vi "main OP300.vi"() -> ()   [LabVIEW 2020]
uses:
  SubVI/OP300ZP_state.ctl
  <userlib>/Alex.vi/FGV.ctl
  <vilib>/QMT/GDataBase for MySQL(tm)/MySQL/public/controls/DateType.ctl
  Documents/GitHub/ZEN-PLUS/OP500/VG/VG_progressBar.vi
  SubVI/CheminDeBase.vi
  <vilib>/Utility/error.llb/Error Cluster From Error Code.vi
  VG/PN.vi
  VG/IS30%.vi
  VG/R.vi
  VG/VG_BT3562.vi
  OP500/VG/VG_ST5520.vi
  Documents/GitHub/ZEN-PLUS/OP300/EN PRODUCTION/OP300-CONTI-AUTO/VG/VG_ARDUINO.vi
  SubVI/VG_HYDRAU.vi
  VG/VG_MX5060.vi
  <vilib>/QMT/GDataBase for MySQL(tm)/MySQL/MySQLConnector.lvclass
panel:
  out "chaîne concaténée":string
  out "MX5060":refnum<visa-resource-name>
  out "ST5520":refnum<visa-resource-name>
  out "Revision":i32=334
  in  "arrêt":bool
  out "BT3562":refnum<visa-resource-name>
  out "Application Directory":path caption="Chemin programme"
  out "Compt":i32
  in  "DERNIER2":bool
  in  "last?":bool
  out "Cluster 2":T1
  out "IS30% ?":bool
  out "BDD":T2
  out "VISA OUT":T3
  out "progression":dbl(slide) scale=0.0..60.0
  out "PN":string
  out "errout":errorcluster={"status"=TRUE, "code"=0, "source"="PCAN_CHANNEL ILLEGAL"}
  out "errout":errorcluster caption="sortie d'erreur"
  out "STOP":bool
  out "TOP":string
  out "DRAW":picture
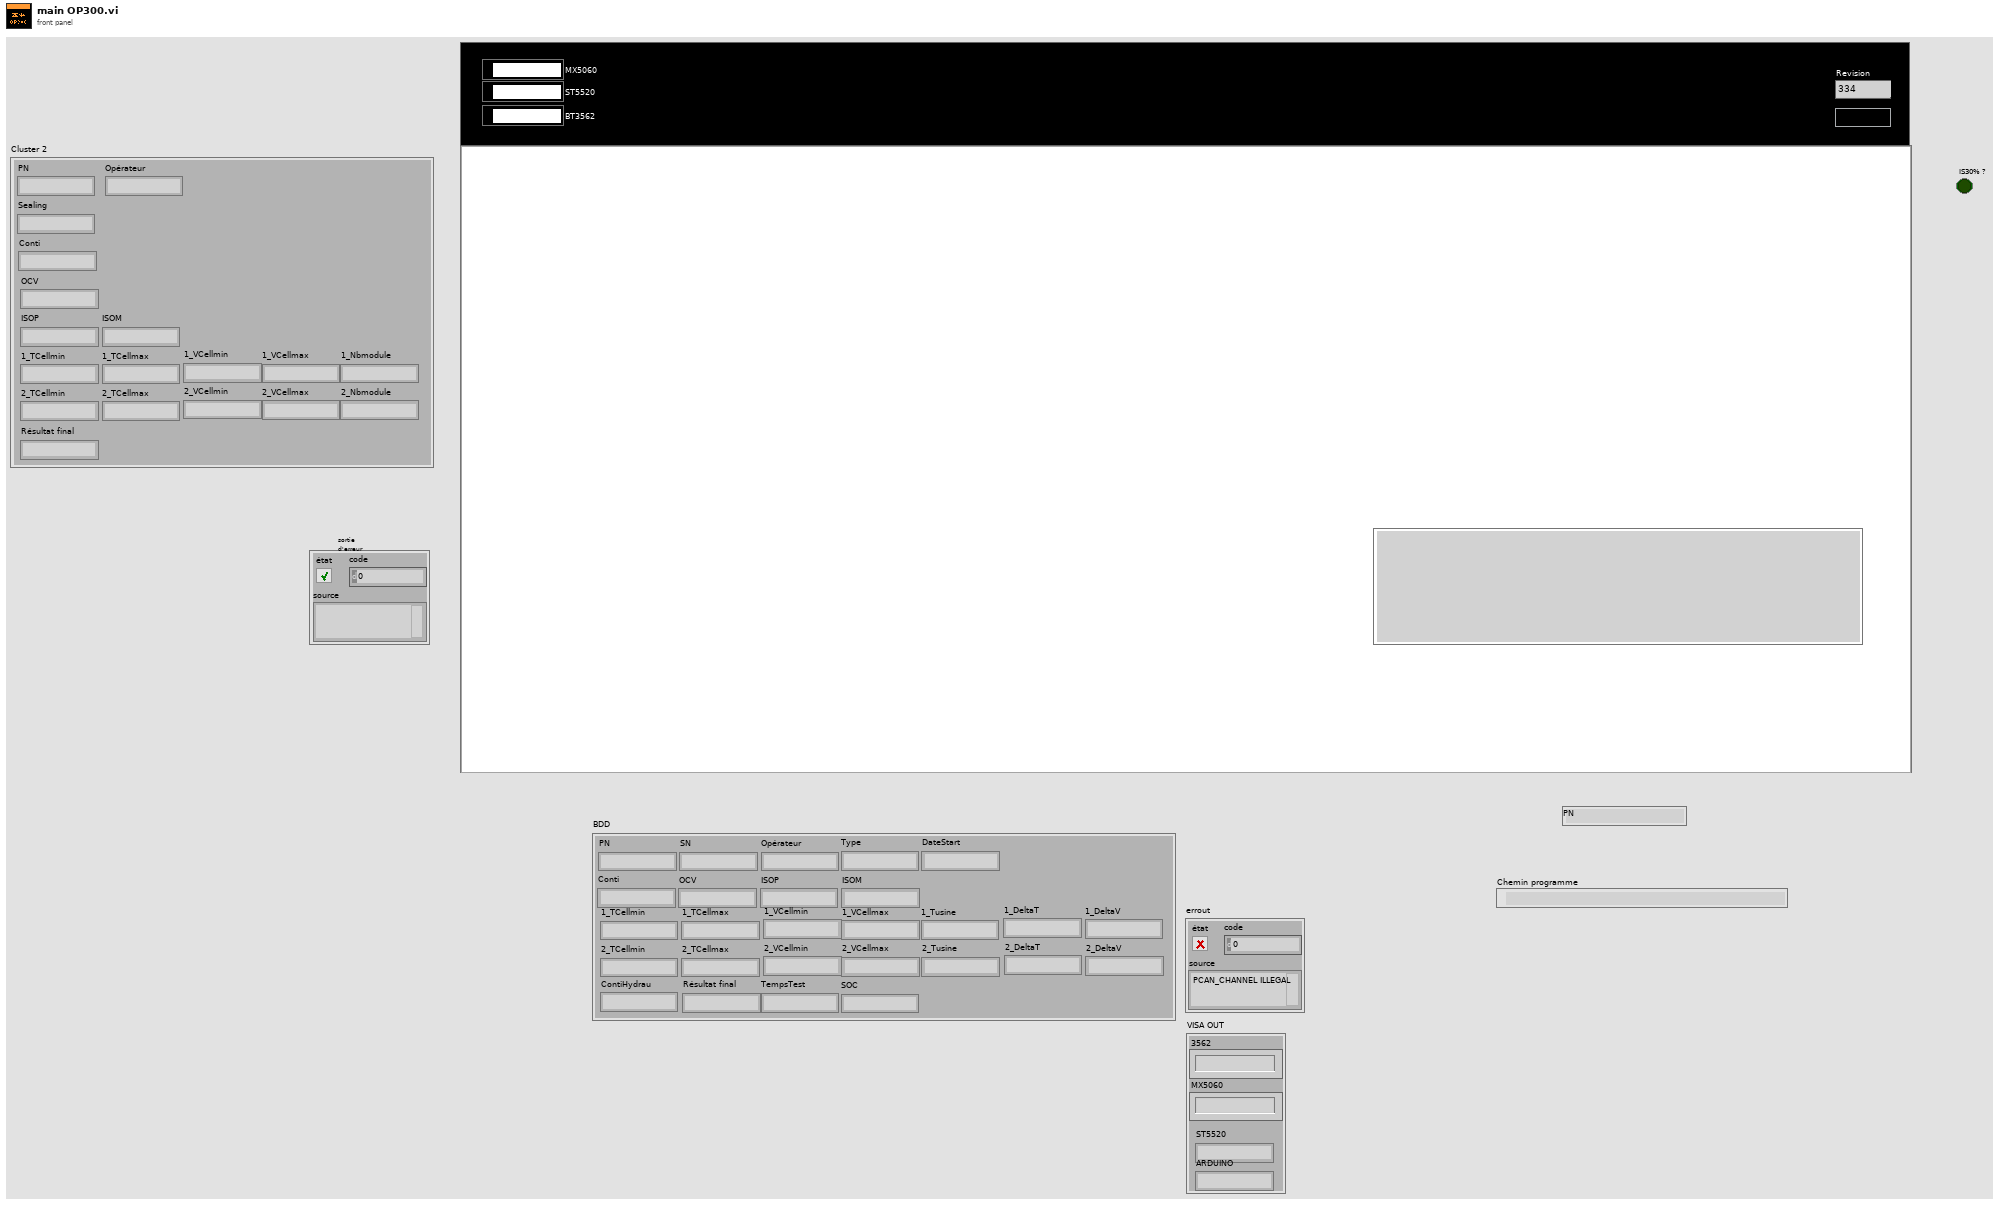
[diagram p1: front panel]
types:
  T1 = cluster{"PN":string, "Opérateur":string, "Sealing":string, "Conti":string, "OCV":string, "ISOP":string, "ISOM":string, "1_TCellmin":string, "1_TCellmax":string, "1_VCellmin":string, "1_VCellmax":string, "1_Nbmodule":string, "2_TCellmin":string, "2_TCellmax":string, "2_VCellmin":string, "2_VCellmax":string, "2_Nbmodule":string, "Résultat final":string}
  T2 = cluster{"PN":string, "SN":string, "Opérateur":string, "Type":string, "DateStart":string, "Conti":string, "OCV":string, "ISOP":string, "ISOM":string, "1_TCellmin":string, "1_TCellmax":string, "1_VCellmin":string, "1_VCellmax":string, "1_Tusine":string, "1_DeltaT":string, "1_DeltaV":string, "2_TCellmin":string, "2_TCellmax":string, "2_VCellmin":string, "2_VCellmax":string, "2_Tusine":string, "2_DeltaT":string, "2_DeltaV":string, "ContiHydrau":string, "Résultat final":string, "TempsTest":string, "SOC":string}
  T3 = cluster{"3562":string, "MX5060":string, "ST5520":string, "ARDUINO":string}
  T4 = cluster{"PN":string, "Sealing":string, "Opérateur":string, "Conti":string, "OCV":string, "ISOP":string, "ISOM":string, "1_TCellmin":string, "1_TCellmax":string, "1_VCellmin":string, "1_VCellmax":string, "1_Nbmodule":string, "2_TCellmin":string, "2_TCellmax":string, "2_VCellmin":string, "2_VCellmax":string, "2_Nbmodule":string, "Résultat final":string, "2_Nbmodule 2":string, "2_VCellmax 2":string, "2_VCellmin 2":string, "2_TCellmax 2":string, "2_TCellmin 2":string, "1_Nbmodule 2":string, "1_VCellmax 2":string, "1_VCellmin 2":string, "1_TCellmax 2":string}
  T5 = cluster{"3562":string, "MX5060":string, "ST5520":string, "ST5520 2":string}
  T6 = typedef "OP300ZP_state.ctl" = enum16{"Null", "Demarrage", "Init", "Scan", "Montage", "Conti", "OCV", "Iso", "Vpack", "DataDyn", "Dessouter", "DataDyn2", "Demontage", "Crash", "Next", "Hydrau", "Sealing", "Comext"}
  T7 = typedef "FGV.ctl" = enum16{"GET", "SET", "RAZ"}
  T8 = typedef "MySQLVIEW.lvlib/MySQLConnector.lvclass/DateType.ctl" = enum16{"DATETIME", "DATE", "TIMESTAMP", "TIME", "YEAR (2 digits)", "YEAR (4 digits)"}
  T9 = cluster{"1_TCellmin":string, "1_TCellmax":string, "1_VCellmin":string, "1_VCellmax":string, "1_Nbmodule":string, "1_TUsine":string, "1_DeltaT":string, "1_DeltaV":string}
  T10 = typedef "imagedata.ctl" = cluster{"image type":i32, "image depth":i32, "image":u8[], "mask":u8[], "colors":u32[], "Rectangle":cluster{"left":i16, "top":i16, "right":i16, "bottom":i16}}
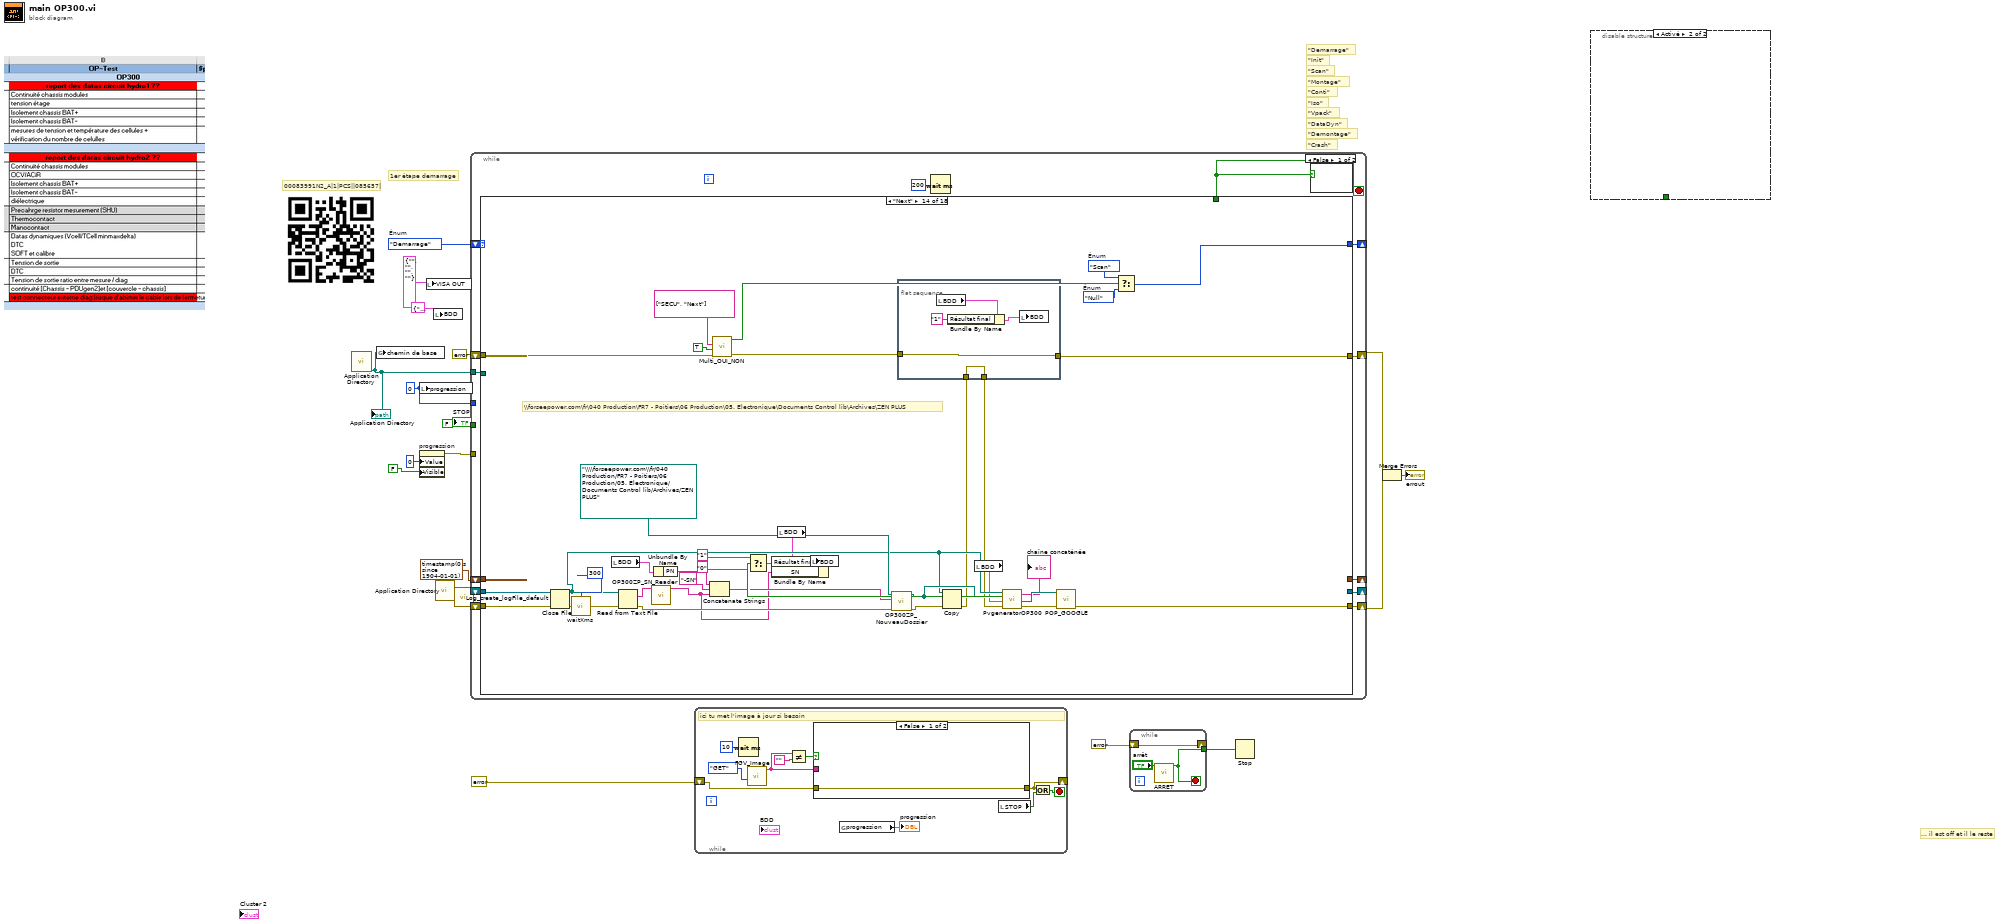
[diagram p0: block diagram]
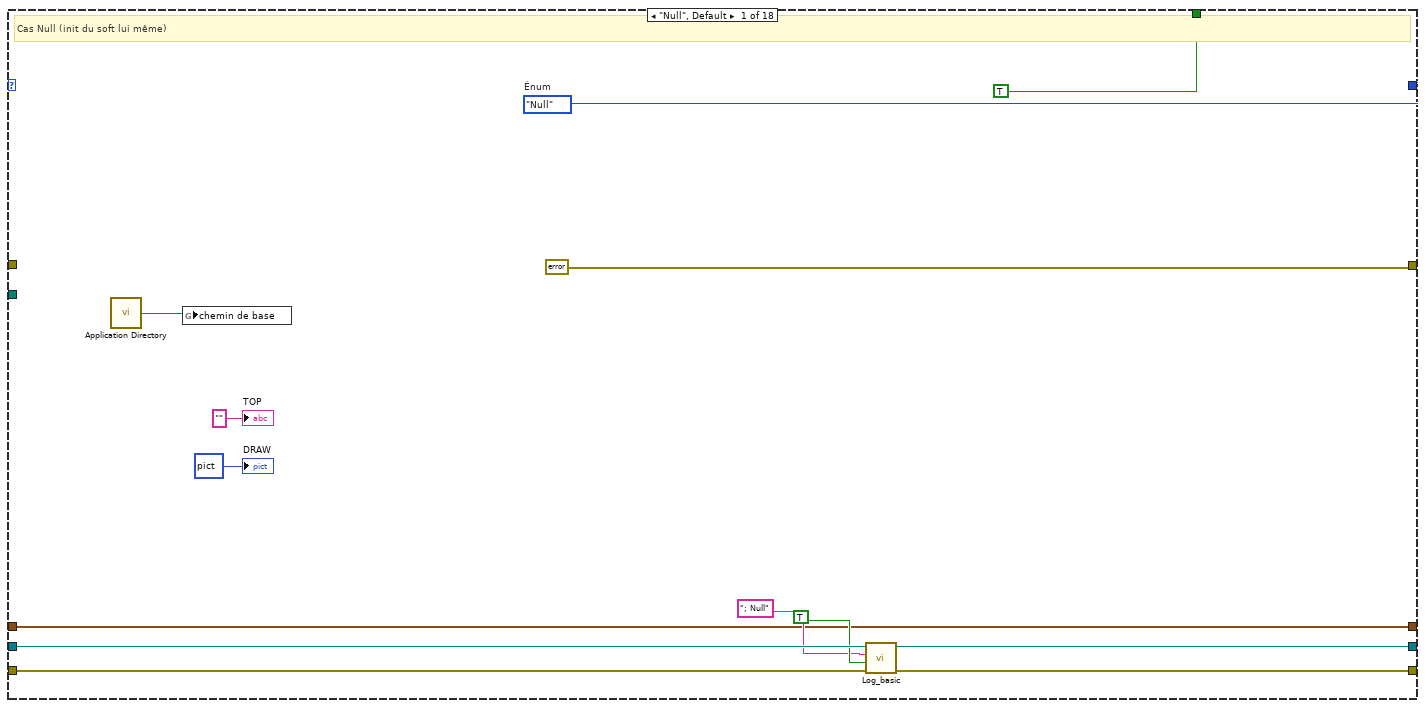
[diagram p2: hidden frame]
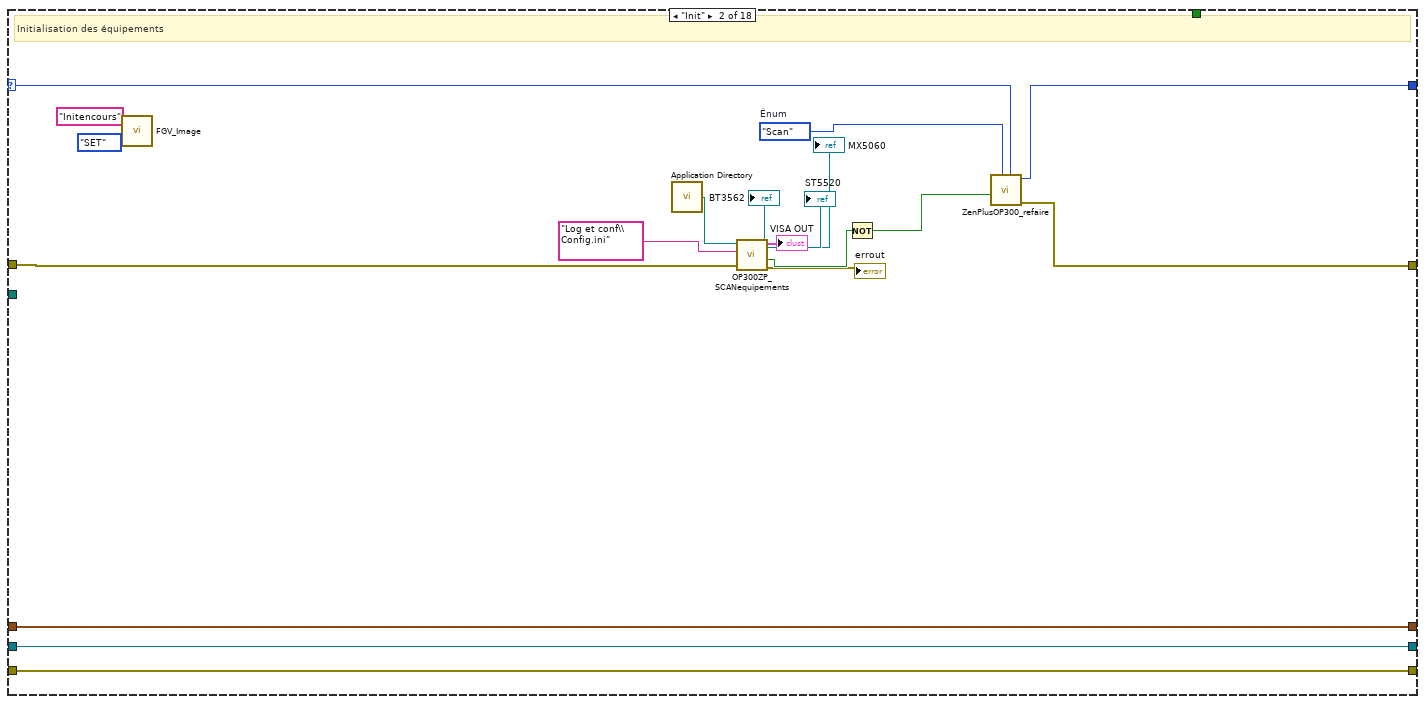
[diagram p3: hidden frame]
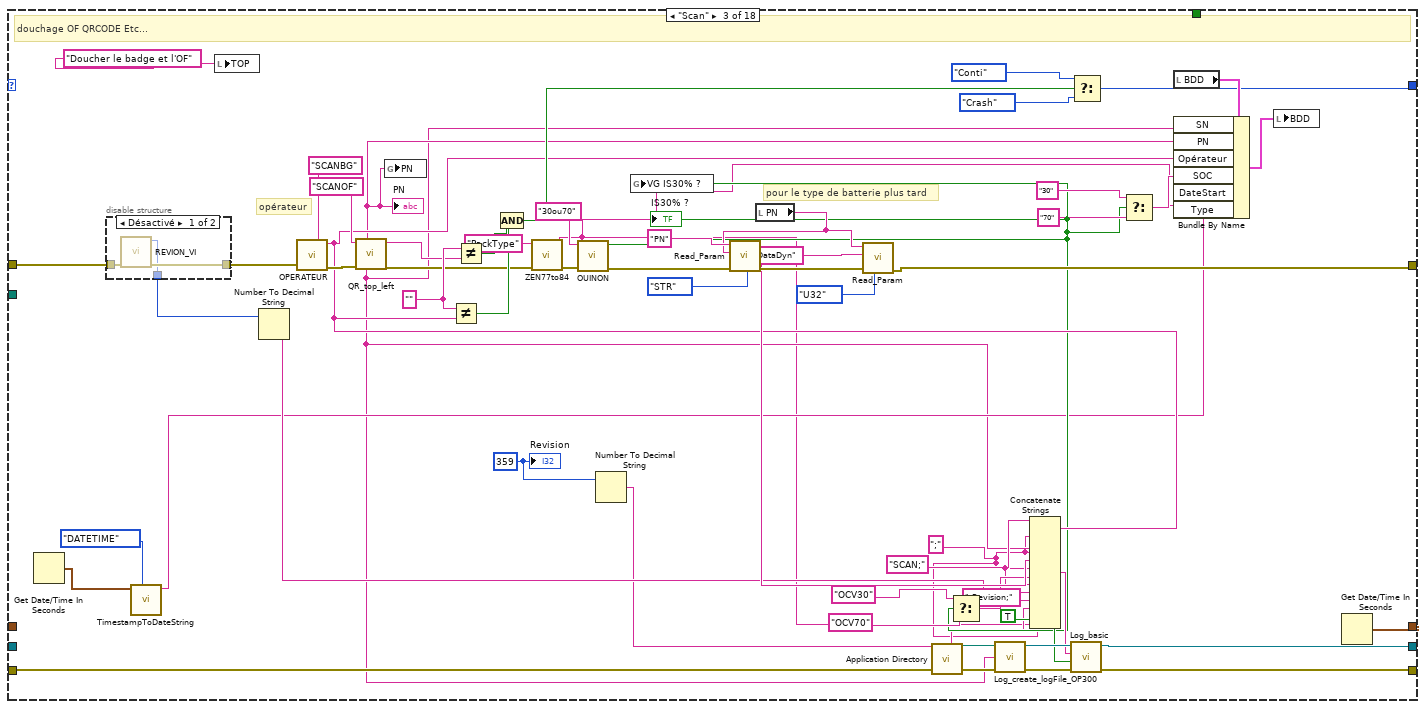
[diagram p4: hidden frame]
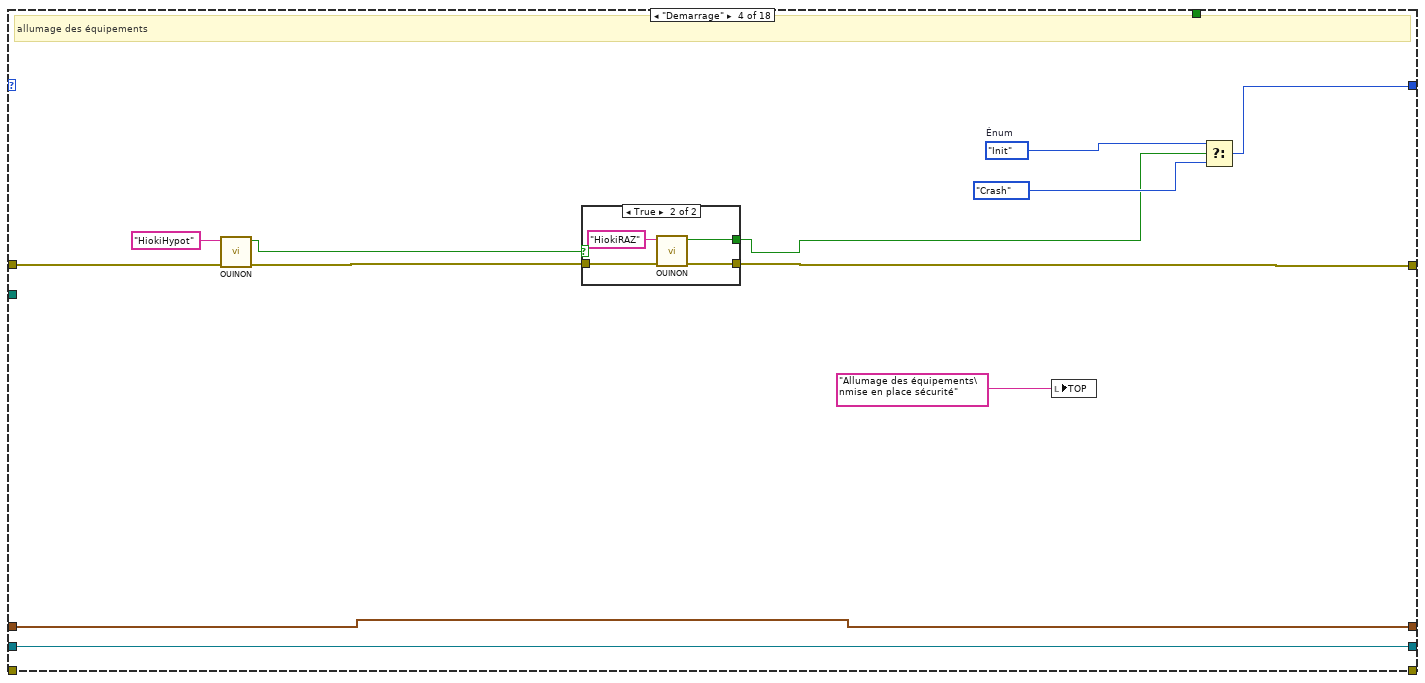
[diagram p6: hidden frame]
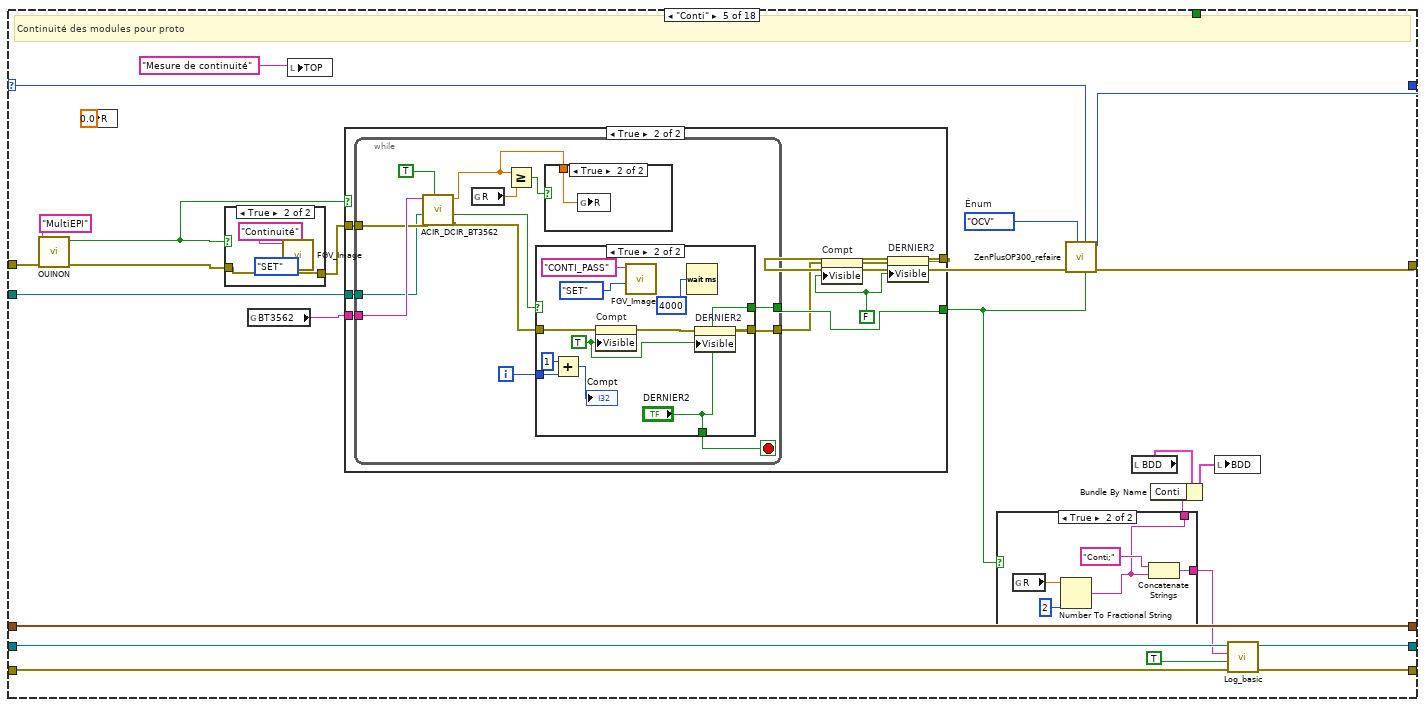
[diagram p8: hidden frame]
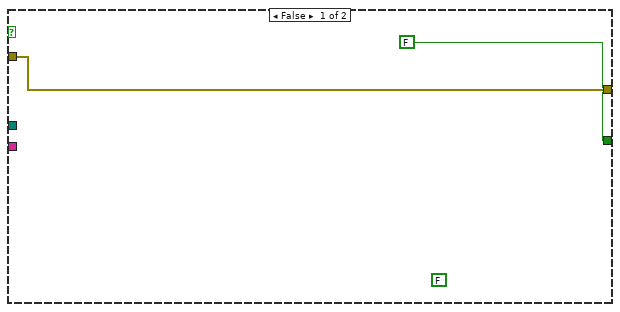
[diagram p10: hidden frame]
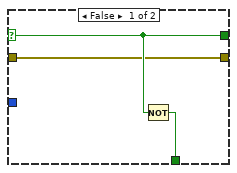
[diagram p11: hidden frame]
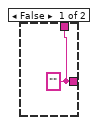
[diagram p13: hidden frame]
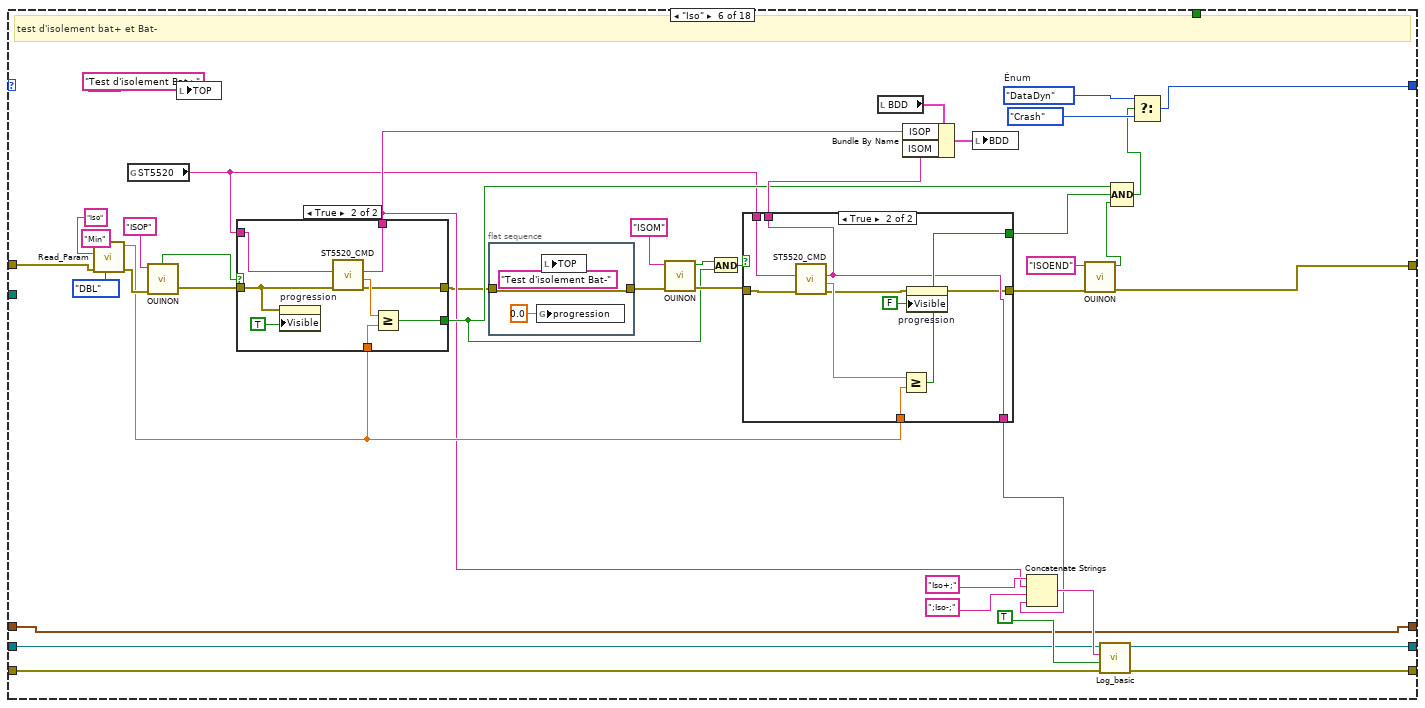
[diagram p14: hidden frame]
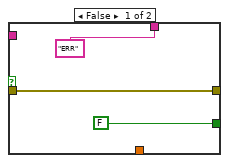
[diagram p15: hidden frame]
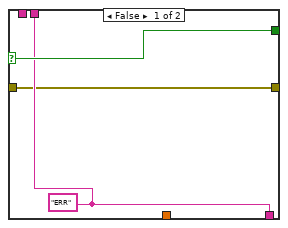
[diagram p16: hidden frame]
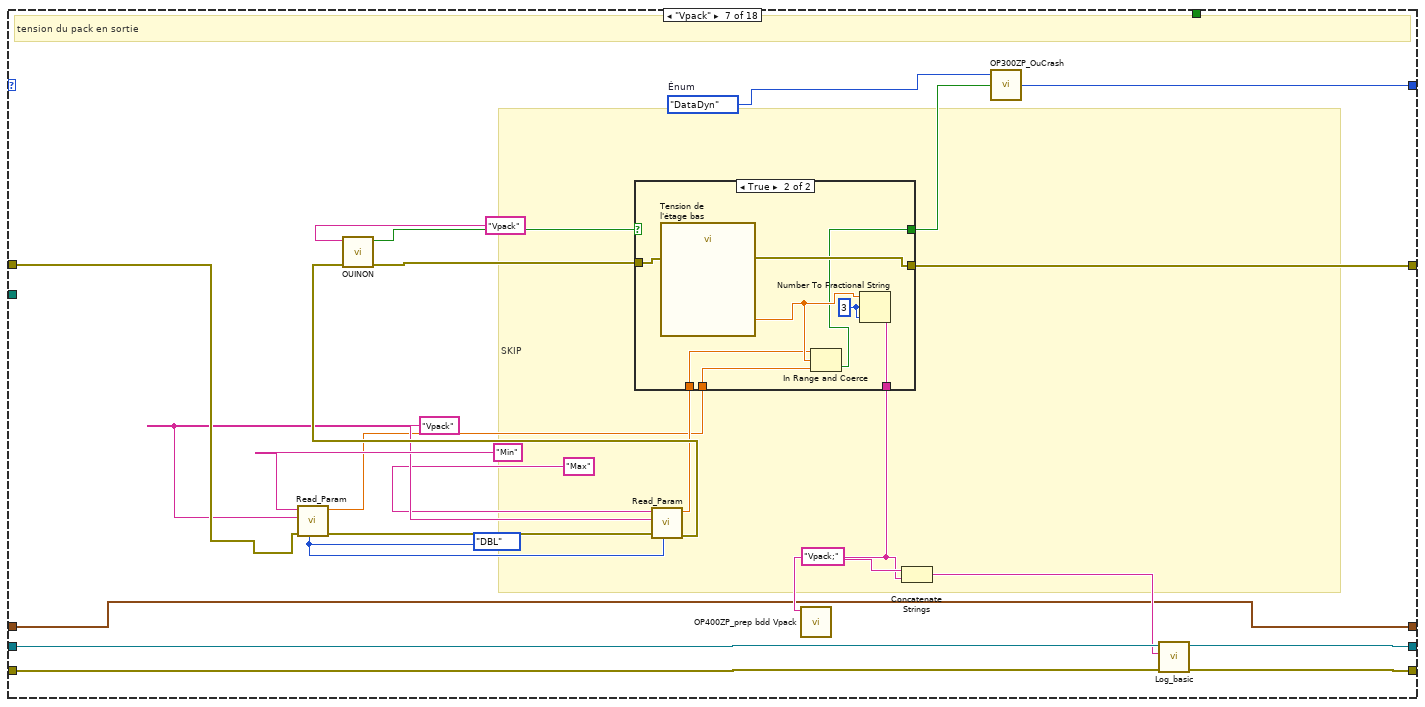
[diagram p17: hidden frame]
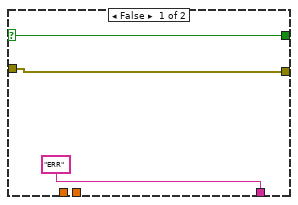
[diagram p18: hidden frame]
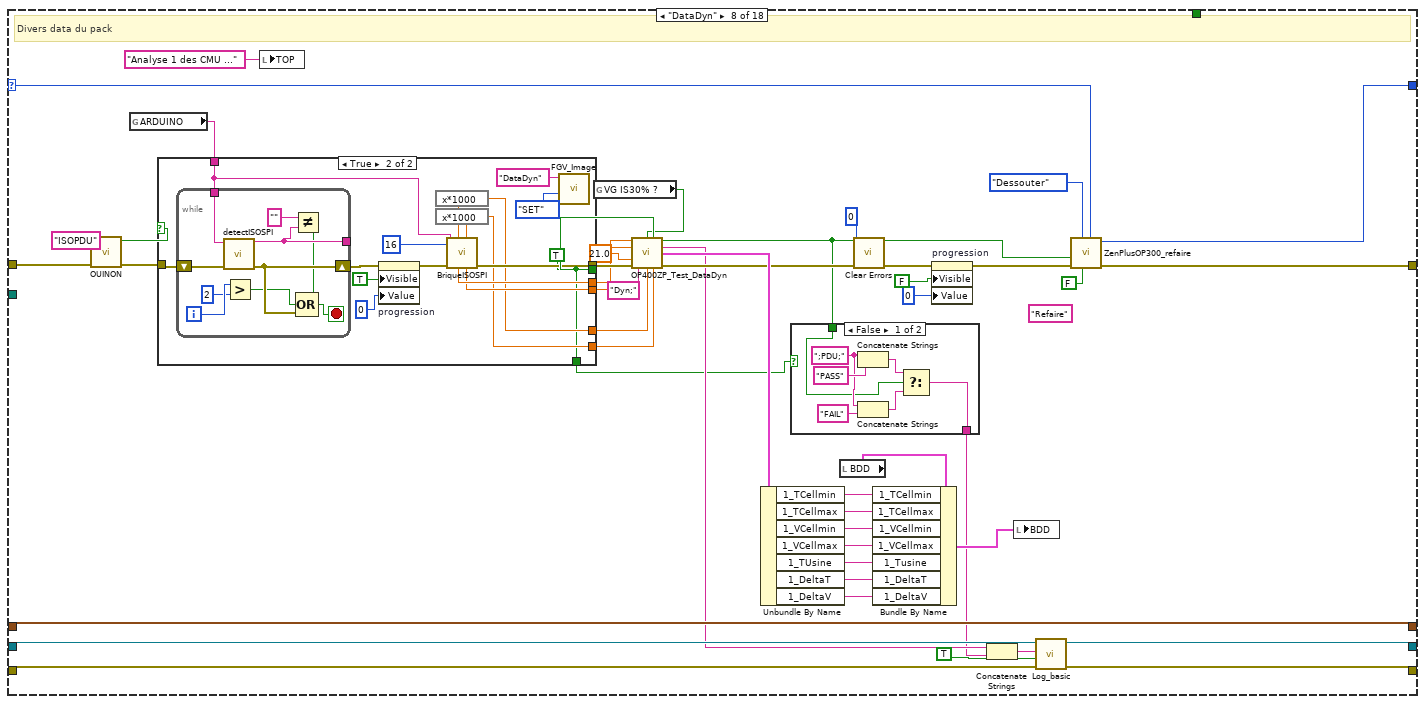
[diagram p19: hidden frame]
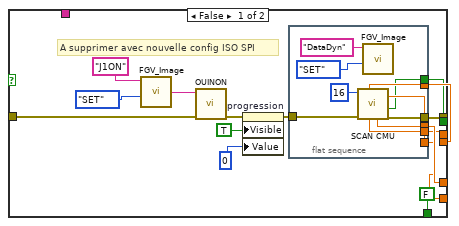
[diagram p20: hidden frame]
diagram:
  w9 = u8 0 ("progression")
  w10 = OP300ZP_state."Demarrage"  # Énum
  w16 = FALSE ("STOP")
  # "00083991N2_A|1|PCS||085657|"
  # "1er étape demarrage"
  # "\"Crash\""
  # "\"Demontage\""
  # "\"DataDyn\""
  # "\"Iso\""
  # "\"Montage\""
  # "\"Scan\""
  # "\"Init\""
  # "\"Demarrage\""
  # "\"Conti\""
  # "\"Vpack\""
  # "... il est off et il le reste"
  n1 = call <vilib>:"Application Directory.vi"() -> ("Application Directory"=w15:path)
  "Application Directory" <- w15
  n2 = global write "CheminDeBase.vi" "chemin de base"(w15) -> ()
  n3 = property on="progression" class="Slide (strict)"("Value"=u8 0 ("progression"), "Visible"=FALSE) -> (error out=w7:errorcluster)  [unwired: 2 in, 1 out]
  n4 = local write "progression"(w9) -> ()
  n5 = local write "VISA OUT"(T5 {"3562"="", "MX5060"="", "ST5520"="", "ST5520 2"=""} ("VISA OUT")) -> ()
  n6 = local write "BDD"(T4 {"PN"="0", "Sealing"="0", "Opérateur"="0", "Conti"="0", "OCV"="0", "ISOP"="0", "ISOM"="0", "1_TCellmin"="0", "1_TCellmax"="0", "1_VCellmin"="0", "1_VCellmax"="0", "1_Nbmodule"="0", "2_TCellmin"="0", "2_TCellmax"="0", "2_VCellmin"="0", "2_VCellmax"="0", "2_Nbmodule"="0", "Résultat final"="0", "2_Nbmodule 2"="0", "2_VCellmax 2"="0", "2_VCellmin 2"="0", "2_TCellmax 2"="0", "2_TCellmin 2"="0", "1_Nbmodule 2"="0", "1_VCellmax 2"="0", "1_VCellmin 2"="0", "1_TCellmax 2"="0"} ("Cluster")) -> ()
  n7 = call <vilib>:"Application Directory.vi"() -> ("Application Directory"=w13:path)
  n8 = call "Log_create_logFile_default.vi"("appdir"=w13) -> ("errout"=w14:errorcluster, "Fichier à flux d'octets en sortie"=w17:refnum<file>)  [unwired: 9 in]
  n9 = while {
    shift-right: [w32] -> w19
    shift-left: errorcluster {"status"=FALSE, "code"=0, "source"=""} ("error out") -> [w22]
    shift-right: [w21] -> _
    shift-left: w10 -> [w26]
    shift-right: [w28] -> w18
    shift-left: w14 -> [w31]
    shift-right: [w29] -> _
    shift-left: w17 -> [w30]
    tunnel: w15 -> [w25]
    tunnel: w16 -> [_]
    shift-right: [w23] -> _
    shift-left: timestamp(0 s since 1904-01-01) ("seconds since 1Jan1904") -> [w24]
    tunnel: w9 -> [_]
    tunnel: w7 -> [_]
    stop <- w27 stop-if-true
    n10 = case shown="\"Next\"" w26 {
      selector: w26 -> [_ w61 _ _ w165 _ _ w363 _ w500 _ _ _ _ w683 w764 w807 w861]
      tunnel: w22 -> [_ w50 w84 w139 w151 w231 w301 w340 w439 w466 w576 w586 w593 w649 w702 w770 w803 w855]
      tunnel: [errorcluster {"status"=FALSE, "code"=0, "source"=""} ("errin") w62 w106 w130 w166 w239 w305 w345 w446 w476 w575 w585 w592 w636 w705 w762 w806 w867] -> w32
      tunnel: w31 -> [w42 w65 w121 _ w171 w250 w310 w367 w438 w497 w573 w587 w615 w668 w707 w769 w811 w870]
      tunnel: w30 -> [w43 w64 _ w140 w170 w249 w309 w368 w436 w499 w574 w588 w616 w669 w706 w767 w810 w872]
      tunnel: [w40 w64 w123 w140 w169 w248 w308 w365 w436 w495 w574 w588 _ _ w685 w766 w809 w868] -> w29
      tunnel: [w41 w65 w124 _ w168 w251 w307 w366 w438 w496 w573 w587 w607 w639 w687 w768 w808 w869] -> w28
      tunnel: [TRUE _ _ _ _ _ _ _ _ _ _ FALSE w617 _ _ _ _ _] -> w27
      tunnel: w25 -> [_ _ _ _ w147 _ _ _ _ _ _ _ _ _ _ _ w805 _]
      tunnel: w24 -> [w36 w63 _ w138 w167 w245 w289 w364 w437 w498 w572 w584 _ _ w704 w765 w800 w871]
      tunnel: [w36 w63 w112 w138 w167 w245 w289 w364 w437 w498 w572 w584 _ _ w704 w765 w801 w871] -> w23
      tunnel: [w34 w51 w86 w131 w157 w230 w287 w350 w435 w481 w567 w579 OP300ZP_state."Crash" w645 w701 w763 w798 w856] -> w21
      frame "Null", Default {
        w34 = OP300ZP_state."Null"  # Énum
        # "Cas Null (init du soft lui même)"
        n11 = call <vilib>:"Application Directory.vi"() -> ("Application Directory"=w46:path)
        n12 = global write "CheminDeBase.vi" "chemin de base"(w46) -> ()
        n13 = call "Log_basic.vi"("errin"=w42, "date?"=TRUE, "chaîne"="; Null", "in"=w43) -> ("sortie d'erreur"=w41:errorcluster, "refnum en sortie"=w40:refnum<file>)  [unwired: 6 in]
        "DRAW" <- picture data[5B] ("DRAW")
        "TOP" <- "" ("TOP")
      }
      frame "Init" {
        w56 = OP300ZP_state."Scan"  # Énum
        # "Initialisation des équipements"
        n14 = call <userlib>:"FGV_Image.vi"("Énum"=FGV."SET", "IN"="Initencours") -> ()  [unwired: 9 in, 1 out]
        n15 = call <vilib>:"Application Directory.vi"() -> ("Application Directory"=w53:path)
        n16 = call "OP300ZP_SCANequipements.vi"("Errin"=w50, "Chaîne"="Log et conf\\Config.ini", "pathin"=w53) -> ("errout 2"=→"errout":errorcluster, "KO?"=w57:bool, "BT3562"=→"BT3562":refnum<visa-resource-name>, "VISA OUT"=→"VISA OUT":T3, "MX5060"=→"MX5060":refnum<visa-resource-name>, "ST5520"=→"ST5520":refnum<visa-resource-name>)  [unwired: 3 in]
        n17 = Not(x=w57) -> (.not. x?=w58:bool)
        n18 = call "ZenPlusOP300_refaire.vi"("refaire"=w61, "casOK"=w56, "test ok ?"=w58) -> ("errout"=w62:errorcluster, "Next"=w51:T6)  [unwired: 7 in]
      }
      frame "Scan" {
        w72 = 359
        w67 = ";" ("chaîne")
        w115 = "" ("x")
        # "pour le type de batterie plus tard"
        # "opérateur"
        # "douchage OF QRCODE Etc..."
        n19 = Get Date/Time In Seconds() -> (seconds since 1Jan1904=w76:timestamp)
        n20 = disable-structure shown="Désactivé" {
          disable-tunnel: w84 -> [w127 w128]
          disable-tunnel: [w126 w128] -> w77
          disable-tunnel: [w125 _] -> w83
          frame Disabled {
            n21 = call "REVION_VI.vi"("ERRIN"=w127) -> ("ERROUT"=w126:errorcluster, "N° Révision"=w125:u32)  [unwired: 9 in]
          }
          frame Enabled {
          }
        }
        n22 = call <vilib>:"TimestampToDateString.vi"("dateType"=DateType."DATETIME", "timestamp in"=w76) -> ("dateString"=w75:string)  [unwired: 8 in, 1 out]
        n23 = local write "TOP"("Doucher le badge et l'OF" ("TOP")) -> ()
        n24 = Number To Decimal String(number=w83) -> (decimal integer string=w82:string)  [unwired: 1 in]
        n25 = call "OPERATEUR.vi"("errin"=w77, "IN"="SCANBG") -> ("error out"=w111:errorcluster, "Dataout"=w93:string)  [unwired: 8 in]
        n26 = call <userlib>:"QR_top_left.vi"("errin"=w111, "image"="SCANOF") -> ("error out"=w85:errorcluster, "Réponse"=w109:string, "SN"=w68:string, "PN"=w87:string)  [unwired: 5 in, 1 out]
        "PN" <- w87
        n27 = global write "PN.vi" "PN"(w87) -> ()
        n28 = Not Equal?(x=w115, y=w93) -> (x != y?=w113:bool)
        n29 = Not Equal?(x=w115, y=w109) -> (x != y?=w114:bool)
        n30 = Compound Arithmetic op=AND ("Opérateur arithmétique")(w114, w113) -> (w99:bool)
        n31 = call <userlib>:"ZEN77to84.vi"("errin"=w85, "image"="PackType") -> ("error out"=w70:errorcluster, "Réponse"=w66:string)  [unwired: 8 in]
        n32 = call <userlib>:"OUINON.vi"("errin"=w70, "image"="30ou70") -> ("error out"=w91:errorcluster, "OUI/NON"=w79:bool)  [unwired: 8 in]
        "IS30% ?" <- w79
        n33 = Number To Decimal String(number=w72) -> (decimal integer string=w71:string)  [unwired: 1 in]
        n34 = global write "IS30%.vi" "VG IS30% ?"(w79) -> ()
        n35 = local read "PN"() -> (w102:string)
        n36 = call <userlib>:"Read_Param.vi"("Énum"=enum16{"STR", "DBL", "U32"}."STR", "errin"=w91, "section"=w102, "key"="PN") -> ("error out"=w105:errorcluster, "str"=w101:string)  [unwired: 3 in, 3 out]
        n37 = call <userlib>:"Read_Param.vi"("Énum"=enum16{"STR", "DBL", "U32"}."U32", "errin"=w105, "section"="DataDyn", "key"=w102) -> ("error out"=w106:errorcluster)  [unwired: 3 in, 4 out]
        n38 = call <vilib>:"Application Directory.vi"() -> ("Application Directory"=w122:path)
        n39 = Select ("Sélectionner")(t="OCV30" ("section"), s=w79, f="OCV70" ("section")) -> (s? t:f=w88:string)
        n40 = call "Log_create_logFile_OP300.vi"("errin"=w121, "toute l'expression"=w68, "Application Directory"=w122) -> ("sortie d'erreur"=w119:errorcluster, "Fichier à flux d'octets en sortie"=w120:refnum<file>)  [unwired: 7 in]
        n41 = Concatenate Strings("SCAN;" ("chaîne"), w93, w67, w68, w67, w101, w67, w88, w67, w82, ";Revision;" ("string"), w71, w67, w66) -> (w117:string)
        n42 = call "Log_basic.vi"("errin"=w119, "date?"=TRUE, "chaîne"=w117, "in"=w120) -> ("sortie d'erreur"=w124:errorcluster, "refnum en sortie"=w123:refnum<file>)  [unwired: 6 in]
        n43 = Select ("Sélectionner")(t=OP300ZP_state."Conti" ("Énum"), s=w99, f=OP300ZP_state."Crash" ("cas faux")) -> (s? t:f=w86:T6)
        n44 = Select(t="30", s=w79, f="70") -> (s? t:f=w78:string)
        n45 = local read "BDD"() -> (w95:T2)
        n46 = Bundle By Name(cluster=w95, "SN"=w68, "PN"=w87, "Opérateur"=w93, "SOC"=w78, "DateStart"=w75, "Type"=w66) -> (w94:T2)
        n47 = local write "BDD"(w94) -> ()
        n48 = Get Date/Time In Seconds() -> (seconds since 1Jan1904=w112:timestamp)
        "Revision" <- w72
      }
      frame "Demarrage" {
        w133 = OP300ZP_state."Init"  # Énum
        # "allumage des équipements"
        n49 = call <userlib>:"OUINON.vi"("errin"=w139, "image"="HiokiHypot") -> ("error out"=w136:errorcluster, "OUI/NON"=w135:bool)  [unwired: 8 in]
        n50 = case shown="True" w135 {
          selector: w135 -> [w142 _]
          tunnel: [w142 w146] -> w129
          tunnel: [w141 w145] -> w130
          tunnel: w136 -> [w141 w143]
          frame False {
          }
          frame True {
            n51 = call <userlib>:"OUINON.vi"("errin"=w143, "image"="HiokiRAZ" ("IN")) -> ("error out"=w145:errorcluster, "OUI/NON"=w146:bool)  [unwired: 8 in]
          }
        }
        n52 = local write "TOP"("Allumage des équipements\nmise en place sécurité" ("TOP")) -> ()
        n53 = Select ("Sélectionner")(t=w133, s=w129, f=OP300ZP_state."Crash" ("cas faux")) -> (s? t:f=w131:T6)
      }
      frame "Conti" {
        w161 = OP300ZP_state."OCV"  # Énum
        # "Continuité des modules pour proto"
        n54 = call <userlib>:"OUINON.vi"("errin"=w151, "image"="MultiEPI") -> ("error out"=w150:errorcluster, "OUI/NON"=w148:bool)  [unwired: 8 in]
        n55 = global write "R.vi" "R"(0.0 ("R")) -> ()
        n56 = case shown="True" w148 {
          tunnel: [w172 w173] -> w149
          tunnel: w150 -> [w172 w173]
          frame False {
          }
          frame True {
            n57 = call <userlib>:"FGV_Image.vi"("Énum"=FGV."SET", "IN"="Continuité") -> ()  [unwired: 9 in, 1 out]
          }
        }
        n58 = global read "VG_BT3562.vi" "BT3562"() -> (w153:string)
        n59 = local write "TOP"("Mesure de continuité" ("TOP")) -> ()
        n60 = case shown="True" w148 {
          tunnel: w153 -> [_ w185]
          tunnel: w149 -> [w177 w184]
          tunnel: [w177 w182] -> w159
          tunnel: [FALSE ("OUI/NON") w183] -> w158
          tunnel: w147 -> [_ w178]
          frame False {
            (unwired) FALSE
          }
          frame True {
            w179 = FALSE ("Visible")
            n61 = while {
              tunnel: w185 -> [w198]
              tunnel: w184 -> [w197]
              tunnel: [w195] -> w181
              tunnel: [w190] -> w183
              tunnel: w178 -> [w186]
              i -> [w194]
              stop <- w189 stop-if-true
              n62 = call <userlib>:"ACIR_DCIR_BT3562.vi"("juste R?"=TRUE, "errin"=w197, "chemin de base"=w186, "VISAin"=w198) -> ("errout"=w188:errorcluster, "OK?"=w196:bool, "R"=w191:dbl)  [unwired: 2 in, 3 out]
              n63 = global read "R.vi" "R"() -> (w193:dbl)
              n64 = Greater Or Equal?(x=w191, y=w193) -> (x >= y?=w192:bool)
              n65 = case shown="True" w196 {
                selector: w196 -> [w201 _]
                tunnel: w188 -> [w199 w208]
                tunnel: [w199 w204] -> w195
                tunnel: [w200 "DERNIER2"] -> w189
                tunnel: w194 -> [_ w210]
                tunnel: [w201 "DERNIER2"] -> w190
                frame False {
                  n66 = Not(x=w201) -> (.not. x?=w200:bool)
                }
                frame True {
                  w202 = TRUE ("Visible")
                  n67 = Add(x=1, y=w210) -> (x+y=→"Compt":i32)
                  n68 = property on="Compt" class="DigNum (strict)"(error in=w208, "Visible"=w202) -> (error out=w205:errorcluster)  [unwired: 1 in, 1 out]
                  n69 = call <userlib>:"FGV_Image.vi"("Énum"=FGV."SET", "IN"="CONTI_PASS") -> ()  [unwired: 9 in, 1 out]
                  n70 = Wait (ms)(milliseconds to wait=u32 4000 ("attente (ms)")) -> ()  [unwired: 1 out]
                  n71 = property on="DERNIER2" class="Bool"(error in=w205, "Visible"=w202) -> (error out=w204:errorcluster)  [unwired: 1 in, 1 out]
                }
              }
              n72 = case shown="True" w192 {
                tunnel: w191 -> [_ w213]
                frame False {
                }
                frame True {
                  n73 = global write "R.vi" "R"(w213) -> ()
                }
              }
            }
            n74 = property on="Compt" class="DigNum (strict)"(error in=w181, "Visible"=w179) -> (error out=w180:errorcluster)  [unwired: 1 in, 1 out]
            n75 = property on="DERNIER2" class="Bool"(error in=w180, "Visible"=w179) -> (error out=w182:errorcluster)  [unwired: 1 in, 1 out]
          }
        }
        n76 = case shown="True" w158 {
          tunnel: [w214 w216] -> w164
          tunnel: [w214 w215] -> w154
          frame False {
            w214 = ""
          }
          frame True {
            n77 = global read "R.vi" "R"() -> (w218:dbl)
            n78 = Number To Fractional String(number=w218, precision (6)=i16 2 ("précision (6)")) -> (F-format string=w215:string)  [unwired: 2 in]
            n79 = Concatenate Strings("Conti;" ("chaîne"), w215) -> (w216:string)
          }
        }
        n80 = call "ZenPlusOP300_refaire.vi"("refaire"=w165, "casOK"=w161, "errin"=w159, "test ok ?"=w158) -> ("errout"=w166:errorcluster, "Next"=w157:T6)  [unwired: 6 in]
        n81 = local read "BDD"() -> (w156:T2)
        n82 = Bundle By Name(cluster=w156, "Conti"=w154) -> (w155:T2)
        n83 = local write "BDD"(w155) -> ()
        n84 = call "Log_basic.vi"("errin"=w171, "date?"=TRUE, "chaîne"=w164, "in"=w170) -> ("sortie d'erreur"=w168:errorcluster, "refnum en sortie"=w169:refnum<file>)  [unwired: 6 in]
      }
      frame "Iso" {
        w244 = OP300ZP_state."DataDyn"  # Énum
        # "test d'isolement bat+ et Bat-"
        n85 = call <userlib>:"Read_Param.vi"("Énum"=enum16{"STR", "DBL", "U32"}."DBL", "errin"=w231, "section"="Iso", "key"="Min") -> ("error out"=w254:errorcluster, "dbl"=w229:dbl)  [unwired: 3 in, 3 out]
        n86 = global read "VG_ST5520.vi" "ST5520"() -> (w222:string)
        n87 = call <userlib>:"OUINON.vi"("errin"=w254, "image"="ISOP" ("IN")) -> ("error out"=w228:errorcluster, "OUI/NON"=w223:bool)  [unwired: 8 in]
        n88 = local write "TOP"("Test d'isolement Bat+" ("TOP")) -> ()
        n89 = case shown="True" w223 {
          tunnel: w229 -> [_ w270]
          tunnel: w228 -> [w262 w264]
          tunnel: [w262 w269] -> w221
          tunnel: [FALSE w268] -> w226
          tunnel: ["ERR" ("DATA OUT") w267] -> w224
          tunnel: w222 -> [_ w266]
          frame False {
          }
          frame True {
            n90 = property on="progression" class="Slide (strict)"(error in=w264, "Visible"=TRUE) -> ()  [unwired: 1 in, 2 out]
            n91 = call "ST5520_CMD.vi"("errin"=w264, "VISA"=w266) -> ("errout"=w269:errorcluster, "DATA FINAL FLT"=w271:dbl, "DATA OUT"=w267:string)  [unwired: 6 in, 1 out]
            n92 = Greater Or Equal?(x=w271, y=w270) -> (x >= y?=w268:bool)
          }
        }
        n93 = flat-sequence {
          tunnel: w221 -> [w273]
          tunnel: [w273] -> w233
          frame #0 {
            n94 = global write "VG_progressBar.vi" "progression"(0.0 ("progression")) -> ()
            n95 = local write "TOP"("Test d'isolement Bat-" ("TOP")) -> ()
          }
        }
        n96 = call <userlib>:"OUINON.vi"("errin"=w233, "image"="ISOM" ("IN")) -> ("error out"=w234:errorcluster, "OUI/NON"=w227:bool)  [unwired: 8 in]
        n97 = And(x=w227, y=w226) -> (x .and. y?=w225:bool)
        n98 = case shown="True" w225 {
          selector: w225 -> [w277 _]
          tunnel: [w275 w279] -> w238
          tunnel: [w276 w282] -> w246
          tunnel: [w277 w283] -> w237
          tunnel: w229 -> [_ w286]
          tunnel: [w276 w282] -> w240
          tunnel: w234 -> [w275 w285]
          tunnel: w222 -> [_ w281]
          frame False {
            w276 = "ERR"
          }
          frame True {
            n99 = call "ST5520_CMD.vi"("errin"=w285, "VISA"=w281) -> ("errout"=w280:errorcluster, "DATA FINAL FLT"=w284:dbl, "DATA OUT"=w282:string)  [unwired: 6 in, 1 out]
            n100 = Greater Or Equal?(x=w284, y=w286) -> (x >= y?=w283:bool)
            n101 = property on="progression" class="Slide (strict)"(error in=w280, "Visible"=FALSE) -> (error out=w279:errorcluster)  [unwired: 1 in, 1 out]
          }
        }
        n102 = local read "BDD"() -> (w242:T2)
        n103 = Bundle By Name(cluster=w242, "ISOP"=w224, "ISOM"=w240) -> (w241:T2)
        n104 = local write "BDD"(w241) -> ()
        n105 = Concatenate Strings("Iso+;" ("chaîne"), w224, ";Iso-;" ("chaîne"), w246) -> (w259:string)
        n106 = call <userlib>:"OUINON.vi"("errin"=w238, "image"="ISOEND") -> ("error out"=w239:errorcluster, "OUI/NON"=w236:bool)  [unwired: 8 in]
        n107 = call "Log_basic.vi"("errin"=w250, "date?"=TRUE, "chaîne"=w259, "in"=w249) -> ("sortie d'erreur"=w251:errorcluster, "refnum en sortie"=w248:refnum<file>)  [unwired: 6 in]
        n108 = Compound Arithmetic op=AND ("Opérateur arithmétique")(w226, w237, w236) -> (w235:bool)
        n109 = Select ("Sélectionner")(t=w244, s=w235, f=OP300ZP_state."Crash" ("cas faux")) -> (s? t:f=w230:T6)
      }
      frame "Vpack" {
        w288 = OP300ZP_state."DataDyn"  # Énum
        w297 = enum16{"STR", "DBL", "U32"}."DBL" ("Énum")
        w299 = "Vpack" ("section")
        # "SKIP"
        # "tension du pack en sortie"
        n110 = call <userlib>:"Read_Param.vi"("Énum"=w297, "errin"=w301, "section"=w299, "key"="Min") -> ("error out"=w302:errorcluster, "dbl"=w295:dbl)  [unwired: 3 in, 3 out]
        n111 = call <userlib>:"Read_Param.vi"("Énum"=w297, "errin"=w302, "section"=w299, "key"="Max") -> ("error out"=w300:errorcluster, "dbl"=w296:dbl)  [unwired: 3 in, 3 out]
        n112 = call <userlib>:"OUINON.vi"("errin"=w300, "image"="Vpack" ("IN")) -> ("error out"=w304:errorcluster, "OUI/NON"=w292:bool)  [unwired: 8 in]
        n113 = case shown="True" w292 {
          selector: w292 -> [w311 _]
          tunnel: w304 -> [w313 w321]
          tunnel: [w313 w318] -> w305
          tunnel: ["ERR" w319] -> w290
          tunnel: [w311 w316] -> w291
          tunnel: w296 -> [_ w314]
          tunnel: w295 -> [_ w315]
          frame False {
          }
          frame True {
            w320 = i16 3 ("largeur (-)")
            n114 = call "Tension de l'étage bas"("error in (no error)"=w321) -> ("Vpack"=w317:dbl, "error out"=w318:errorcluster)  [unwired: 16 in, 1 out]
            n115 = In Range and Coerce(upper limit=w314, x=w317, lower limit=w315) -> (In Range?=w316:bool)  [unwired: 1 out]
            n116 = Number To Fractional String(number=w317, width (-)=w320, precision (6)=w320) -> (F-format string=w319:string)  [unwired: 1 in]
          }
        }
        n117 = call "OP400ZP_prep bdd Vpack.vi"("OCV"=w290) -> ()  [unwired: 10 in, 1 out]
        n118 = Concatenate Strings("Vpack;" ("chaîne"), w290) -> (w293:string)
        n119 = call "OP300ZP_OuCrash.vi"("Booléen"=w291, "in"=w288) -> ("OUT"=w287:T6)  [unwired: 1 in]
        n120 = call "Log_basic.vi"("errin"=w310, "chaîne"=w293, "in"=w309) -> ("sortie d'erreur"=w307:errorcluster, "refnum en sortie"=w308:refnum<file>)  [unwired: 7 in]
      }
      frame "DataDyn" {
        (unwired) "Refaire" ("image")
        # "Divers data du pack"
        n121 = call <userlib>:"OUINON.vi"("errin"=w340, "image"="ISOPDU") -> ("error out"=w339:errorcluster, "OUI/NON"=w328:bool)  [unwired: 8 in]
        n122 = global read "VG_ARDUINO.vi" "ARDUINO"() -> (w322:string)
        n123 = case shown="True" w328 {
          tunnel: w339 -> [w383 w400]
          tunnel: [w382 w406] -> w337
          tunnel: [w381 w405] -> w336
          tunnel: [w380 w404] -> w335
          tunnel: [w379 w407] -> w334
          tunnel: [w378 w408] -> w333
          tunnel: [w377 w403] -> w332
          tunnel: [FALSE ("MCU") w403] -> w325
          tunnel: w322 -> [_ w394]
          frame False {
            # "A supprimer avec nouvelle config ISO SPI"
            n124 = call <userlib>:"FGV_Image.vi"("Énum"=FGV."SET", "IN"="J1ON") -> ("OUT"=w371:string)  [unwired: 9 in]
            n125 = call <userlib>:"OUINON.vi"("errin"=w383, "image"=w371) -> ("error out"=w370:errorcluster)  [unwired: 8 in, 1 out]
            n126 = property on="progression" class="Slide (strict)"(error in=w370, "Visible"=TRUE, "Value"=u8 0 ("progression")) -> (error out=w375:errorcluster)  [unwired: 1 in, 1 out]
            n127 = flat-sequence {
              tunnel: [w393] -> w382
              tunnel: [w392] -> w381
              tunnel: [w391] -> w380
              tunnel: [w390] -> w379
              tunnel: [w389] -> w378
              tunnel: [w388] -> w377
              tunnel: w375 -> [w387]
              frame #0 {
                n128 = call <userlib>:"SCAN CMU.vi"("errin"=w387, "Nb modules"=i16 16) -> ("errout"=w393:errorcluster, "# température + #tension OK?"=w388:bool, "Vmin"=w392:dbl, "Vmax"=w391:dbl, "Tmin"=w389:dbl, "Tmax"=w390:dbl)  [unwired: 4 out]
                n129 = call <userlib>:"FGV_Image.vi"("Énum"=FGV."SET", "IN"="DataDyn") -> ()  [unwired: 9 in, 1 out]
              }
            }
          }
          frame True {
            w403 = TRUE ("MCU")
            n130 = while {
              tunnel: [w417] -> _
              shift-right: [w418] -> w397
              shift-left: w400 -> [w420]
              tunnel: w394 -> [w411]
              i -> [w414]
              stop <- w419 stop-if-true
              n131 = call "detectISOSPI.vi"("errin"=w420, "VISA"=w411) -> ("sortie d'erreur"=w418:errorcluster, "cas faux"=w417:string)  [unwired: 8 in]
              n132 = Greater? ("Supérieur ?")(x=w414, y=2) -> (0:w412:bool)
              n133 = Not Equal? ("Différents ?")(x="", y=w417) -> (x != y?=w415:bool)
              n134 = Compound Arithmetic op=OR ("Opérateur arithmétique")(w415, w412, w418) -> (w419:bool)
            }
            n135 = property on="progression" class="Slide (strict)"(error in=w397, "Visible"=TRUE, "Value"=u8 0 ("progression")) -> (error out=w396:errorcluster)  [unwired: 1 in, 1 out]
            n136 = call "BriqueISOSPI.vi"("errin"=w396, "nbmodule"=16, "visain"=w394) -> ("errout"=w406:errorcluster, "TCellmax"=w407:dbl, "VCellmax"=w409:dbl, "TCellmin"=w408:dbl, "VCellmin"=w410:dbl)  [unwired: 1 in, 3 out]
            n137 = expression code="x*1000"(w410) -> (w405:dbl)
            n138 = expression code="x*1000"(w409) -> (w404:dbl)
            n139 = call <userlib>:"FGV_Image.vi"("Énum"=FGV."SET", "IN"="DataDyn") -> ()  [unwired: 9 in, 1 out]
          }
        }
        n140 = local write "TOP"("Analyse 1 des CMU ..." ("TOP")) -> ()
        n141 = global read "IS30%.vi" "VG IS30% ?"() -> (w329:bool)
        n142 = call "OP400ZP_Test_DataDyn.vi"("Tcell Min (°C)"=w333, "is30%?"=w329, "MCU"=w332, "Tcell Max (°C)"=w334, "Température usine (°C)"=21.0, "errin"=w337, "testname"="Dyn;", "Vcell Min (V)"=w336, "Vcell Max (V)"=w335) -> ("pass"=w324:bool, "datalog"=w327:string, "Cluster"=w356:T9, "errout"=w342:errorcluster)  [unwired: 2 in, 1 out]
        n143 = Unbundle By Name(w356) -> ("1_TCellmin"=w355:string, "1_TCellmax"=w354:string, "1_VCellmin"=w353:string, "1_VCellmax"=w352:string, "1_TUsine"=w351:string, "1_DeltaT"=w349:string, "1_DeltaV"=w348:string)
        n144 = case shown="False" w325 {
          tunnel: w324 -> [w422 w434]
          tunnel: [w421 w428] -> w323
          frame False {
            w425 = ";PDU;" ("chaîne")
            n145 = Concatenate Strings(w425, "PASS" ("chaîne")) -> (w427:string)
            n146 = Concatenate Strings(w425, "FAIL" ("chaîne")) -> (w423:string)
            n147 = Select(t=w427, s=w422, f=w423) -> (s? t:f=w421:string)
          }
          frame True {
            w431 = ";ISOSPI;" ("chaîne")
            n148 = Concatenate Strings(w431, "PASS" ("chaîne")) -> (w433:string)
            n149 = Concatenate Strings(w431, "FAIL" ("chaîne")) -> (w429:string)
            n150 = Select(t=w433, s=w434, f=w429) -> (s? t:f=w428:string)
          }
        }
        n151 = local read "BDD"() -> (w358:T2)
        n152 = call <vilib>:"Clear Errors.vi"("error in (no error)"=w342, "specific error code to clear (0: all)"=0) -> ("error out"=w341:errorcluster)  [unwired: 4 in, 1 out]
        n153 = Bundle By Name(cluster=w358, "1_TCellmin"=w355, "1_TCellmax"=w354, "1_VCellmin"=w353, "1_VCellmax"=w352, "1_Tusine"=w351, "1_DeltaT"=w349, "1_DeltaV"=w348) -> (w357:T2)
        n154 = property on="progression" class="Slide (strict)"(error in=w341, "Visible"=FALSE, "Value"=u8 0 ("progression")) -> (error out=w344:errorcluster)  [unwired: 1 in, 1 out]
        n155 = Concatenate Strings(w327, w323) -> (w326:string)
        n156 = local write "BDD"(w357) -> ()
        n157 = call "Log_basic.vi"("errin"=w367, "date?"=TRUE, "chaîne"=w326, "in"=w368) -> ("sortie d'erreur"=w366:errorcluster, "refnum en sortie"=w365:refnum<file>)  [unwired: 6 in]
        n158 = call "ZenPlusOP300_refaire.vi"("refaire"=w363, "Pédale"=FALSE, "casOK"=OP300ZP_state."Dessouter" ("Énum"), "errin"=w344, "test ok ?"=w324) -> ("errout"=w345:errorcluster, "Next"=w350:T6)  [unwired: 5 in]
      }
      frame "Dessouter" {
        n159 = local write "TOP"("Prendre le MODOP DESSOUTER" ("TOP")) -> ()
        n160 = call <userlib>:"FGV_Image.vi"("Énum"=FGV."SET", "IN"="Echangeur") -> ("OUT"=w451:string)  [unwired: 9 in]
        n161 = call <userlib>:"OUINON.vi"("errin"=w439, "image"=w451) -> ("error out"=w447:errorcluster, "OUI/NON"=w444:bool)  [unwired: 8 in]
        n162 = call <userlib>:"FGV_Image.vi"("Énum"=FGV."SET", "IN"="DessouterEnd") -> ("OUT"=w450:string)  [unwired: 9 in]
        n163 = call <userlib>:"OUINON.vi"("errin"=w447, "image"=w450) -> ("error out"=w446:errorcluster, "OUI/NON"=w445:bool)  [unwired: 8 in]
        n164 = Compound Arithmetic op=AND(w444, w445) -> (w443:bool)
        n165 = Select(t=OP300ZP_state."DataDyn2" ("Next"), s=w443, f=OP300ZP_state."Crash" ("cas faux")) -> (s? t:f=w435:T6)
      }
      frame "DataDyn2" {
        n166 = call <userlib>:"OUINON.vi"("errin"=w466, "image"="ISOPDU") -> ("error out"=w469:errorcluster, "OUI/NON"=w467:bool)  [unwired: 8 in]
        n167 = global read "VG_ARDUINO.vi" "ARDUINO"() -> (w454:string)
        n168 = case shown="True" w467 {
          tunnel: w469 -> [w515 w532]
          tunnel: [w514 w538] -> w465
          tunnel: [w513 w537] -> w464
          tunnel: [w512 w536] -> w463
          tunnel: [w511 w539] -> w462
          tunnel: [w510 w540] -> w461
          tunnel: [w509 w535] -> w455
          tunnel: [FALSE ("MCU") w535] -> w460
          tunnel: w454 -> [_ w526]
          frame False {
            # "A supprimer avec nouvelle config ISO SPI"
            n169 = call <userlib>:"FGV_Image.vi"("Énum"=FGV."SET", "IN"="J1ON") -> ("OUT"=w503:string)  [unwired: 9 in]
            n170 = call <userlib>:"OUINON.vi"("errin"=w515, "image"=w503) -> ("error out"=w502:errorcluster)  [unwired: 8 in, 1 out]
            n171 = property on="progression" class="Slide (strict)"(error in=w502, "Visible"=TRUE, "Value"=u8 0 ("progression")) -> (error out=w507:errorcluster)  [unwired: 1 in, 1 out]
            n172 = flat-sequence {
              tunnel: [w525] -> w514
              tunnel: [w524] -> w513
              tunnel: [w523] -> w512
              tunnel: [w522] -> w511
              tunnel: [w521] -> w510
              tunnel: [w520] -> w509
              tunnel: w507 -> [w519]
              frame #0 {
                n173 = call <userlib>:"SCAN CMU.vi"("errin"=w519, "Nb modules"=i16 16) -> ("errout"=w525:errorcluster, "# température + #tension OK?"=w520:bool, "Vmin"=w524:dbl, "Vmax"=w523:dbl, "Tmin"=w521:dbl, "Tmax"=w522:dbl)  [unwired: 4 out]
                n174 = call <userlib>:"FGV_Image.vi"("Énum"=FGV."SET", "IN"="DataDyn") -> ()  [unwired: 9 in, 1 out]
              }
            }
          }
          frame True {
            w535 = TRUE ("MCU")
            n175 = while {
              tunnel: [w549] -> _
              shift-right: [w550] -> w529
              shift-left: w532 -> [w552]
              tunnel: w526 -> [w543]
              i -> [w546]
              stop <- w551 stop-if-true
              n176 = call "detectISOSPI.vi"("errin"=w552, "VISA"=w543) -> ("sortie d'erreur"=w550:errorcluster, "cas faux"=w549:string)  [unwired: 8 in]
              n177 = Greater? ("Supérieur ?")(x=w546, y=2) -> (0:w544:bool)
              n178 = Not Equal? ("Différents ?")(x="", y=w549) -> (x != y?=w547:bool)
              n179 = Compound Arithmetic op=OR ("Opérateur arithmétique")(w547, w544, w550) -> (w551:bool)
            }
            n180 = property on="progression" class="Slide (strict)"(error in=w529, "Visible"=TRUE, "Value"=u8 0 ("progression")) -> (error out=w528:errorcluster)  [unwired: 1 in, 1 out]
            n181 = call "BriqueISOSPI.vi"("errin"=w528, "nbmodule"=16, "visain"=w526) -> ("errout"=w538:errorcluster, "TCellmax"=w539:dbl, "VCellmax"=w541:dbl, "TCellmin"=w540:dbl, "VCellmin"=w542:dbl)  [unwired: 1 in, 3 out]
            n182 = expression code="x*1000"(w542) -> (w537:dbl)
            n183 = expression code="x*1000"(w541) -> (w536:dbl)
            n184 = call <userlib>:"FGV_Image.vi"("Énum"=FGV."SET", "IN"="DataDyn") -> ()  [unwired: 9 in, 1 out]
          }
        }
        n185 = local write "TOP"("Analyse 2 des CMU ..." ("TOP")) -> ()
        n186 = global read "IS30%.vi" "VG IS30% ?"() -> (w482:bool)
        n187 = call "OP400ZP_Test_DataDyn.vi"("Tcell Min (°C)"=w461, "is30%?"=w482, "MCU"=w455, "Tcell Max (°C)"=w462, "Température usine (°C)"=21.0, "errin"=w465, "testname"="Dyn2;", "Vcell Min (V)"=w464, "Vcell Max (V)"=w463) -> ("pass"=w459:bool, "datalog"=w457:string, "Cluster"=w480:T9, "errout"=w471:errorcluster)  [unwired: 2 in, 1 out]
        n188 = case shown="True" w460 {
          tunnel: [w554 w561] -> w456
          tunnel: w459 -> [w553 w560]
          frame False {
            w557 = ";PDU;" ("chaîne")
            n189 = Concatenate Strings(w557, "PASS" ("chaîne")) -> (w559:string)
            n190 = Concatenate Strings(w557, "FAIL" ("chaîne")) -> (w555:string)
            n191 = Select(t=w559, s=w553, f=w555) -> (s? t:f=w554:string)
          }
          frame True {
            w564 = ";ISOSPI;" ("chaîne")
            n192 = Concatenate Strings(w564, "PASS" ("chaîne")) -> (w566:string)
            n193 = Concatenate Strings(w564, "FAIL" ("chaîne")) -> (w562:string)
            n194 = Select(t=w566, s=w560, f=w562) -> (s? t:f=w561:string)
          }
        }
        n195 = call <vilib>:"Clear Errors.vi"("error in (no error)"=w471, "specific error code to clear (0: all)"=0) -> ("error out"=w472:errorcluster)  [unwired: 4 in, 1 out]
        n196 = Unbundle By Name(w480) -> ("1_TCellmin"=w487:string, "1_TCellmax"=w486:string, "1_VCellmin"=w485:string, "1_VCellmax"=w484:string, "1_TUsine"=w479:string, "1_DeltaT"=w478:string, "1_DeltaV"=w477:string)
        n197 = Concatenate Strings(w457, w456) -> (w458:string)
        n198 = property on="progression" class="Slide (strict)"(error in=w472, "Visible"=FALSE, "Value"=u8 0 ("progression")) -> (error out=w470:errorcluster)  [unwired: 1 in, 1 out]
        n199 = local read "BDD"() -> (w489:T2)
        n200 = Bundle By Name(cluster=w489, "2_TCellmin"=w487, "2_TCellmax"=w486, "2_VCellmin"=w485, "2_VCellmax"=w484, "2_Tusine"=w479, "2_DeltaT"=w478, "2_DeltaV"=w477) -> (w488:T2)
        n201 = call "ZenPlusOP300_refaire.vi"("refaire"=w500, "Pédale"=FALSE, "casOK"=OP300ZP_state."Demontage" ("Énum"), "errin"=w470, "test ok ?"=w459) -> ("errout"=w476:errorcluster, "Next"=w481:T6)  [unwired: 5 in]
        n202 = local write "BDD"(w488) -> ()
        n203 = call "Log_basic.vi"("errin"=w497, "date?"=TRUE, "chaîne"=w458, "in"=w499) -> ("sortie d'erreur"=w496:errorcluster, "refnum en sortie"=w495:refnum<file>)  [unwired: 6 in]
      }
      frame "Montage" {
        w570 = OP300ZP_state."Conti"  # Énum
        # "montage du produit sur le banc"
        n204 = local write "TOP"("Montage du pack" ("TOP")) -> ()
        n205 = call <userlib>:"OUINON.vi"("errin"=w576, "image"="Montage" ("IN")) -> ("error out"=w575:errorcluster, "OUI/NON"=w571:bool)  [unwired: 8 in]
        n206 = Select ("Sélectionner")(t=w570, s=w571, f=OP300ZP_state."Crash" ("cas faux")) -> (s? t:f=w567:T6)
      }
      frame "Demontage" {
        w582 = OP300ZP_state."Hydrau"  # Énum
        n207 = call <userlib>:"OUINON.vi"("errin"=w586, "image"="Demontage" ("IN")) -> ("error out"=w585:errorcluster, "OUI/NON"=w583:bool)  [unwired: 8 in]
        n208 = Select ("Sélectionner")(t=w582, s=w583, f=OP300ZP_state."Crash" ("cas faux")) -> (s? t:f=w579:T6)
        n209 = local write "TOP"("Demontage du pack" ("TOP")) -> ()
      }
      frame "Crash" {
        # "\\\\forseepower.com\\fr\\040 Production\\FR7 - Poitiers\\06 Production\\05. Electronique\\Documents Control lib\\Archives\\ZEN PLUS"
        n210 = Close File(refnum=w616, error in=w615) -> (path=w605:path, error out=w609:errorcluster)
        n211 = call <userlib>:"waitXms.vi"("attente (ms)"=u32 300, "errin"=w609) -> ("errout"=w606:errorcluster)  [unwired: 13 in]
        n212 = local read "BDD"() -> (w599:T2)
        n213 = Read from Text File(file (use dialog)=w605, error in=w606) -> (text=w604:string, error out=w602:errorcluster)  [unwired: 2 in, 2 out]
        n214 = call "OP300ZP_SN_Reader.vi"("Fichier txt"=w604) -> ("SN"=w597:string)  [unwired: 10 in]
        n215 = Unbundle By Name(w599) -> ("PN"=w596:string)
        n216 = call <userlib>:"FGV_Image.vi"("Énum"=FGV."SET", "IN"="TeamLeader") -> ()  [unwired: 9 in, 1 out]
        n217 = Concatenate Strings(w596, "-SN" ("chaîne"), w597) -> (w598:string)
        n218 = call "OP300ZP_NouveauDossier.vi"("entrée d'erreur (pas d'erreur)"=w602, "Nom du repertoire (PN SN)"=w598, "Network before adding a new folder"=path "\\\\forseepower.com\\fr/040 Production/FR7 - Poitiers/06 Production/05. Electronique/Documents Control lib/Archives/ZEN PLUS" ("chemin de la cible (utiliser une boîte de dialogue)")) -> ("sortie d'erreur"=w603:errorcluster, "Network after adding a new folder"=w600:path)  [unwired: 7 in]
        n219 = Copy ("Copier")(8:w603, 10:w600, 11:w605) -> (0:w591:errorcluster)  [unwired: 2 in, 2 out]
        n220 = flat-sequence {
          tunnel: w593 -> [w622]
          tunnel: [w622] -> w592
          tunnel: w591 -> [w618]
          tunnel: [w618] -> w590
          frame #0 {
            n221 = local read "BDD"() -> (w621:T2)
            n222 = Bundle By Name(cluster=w621, "Résultat final"="0") -> (w619:T2)
            n223 = local write "BDD"(w619) -> ()
          }
        }
        n224 = call "PvgeneratorOP300.vi"("errin"=w590, "network"=w600, "path in"=w605) -> ("sortie d'erreur"=w612:errorcluster, "network out"=w611:path)  [unwired: 4 in, 3 out]
        n225 = call "POP_GOOGLE.vi"("error in"=w612, "chemin"=w611) -> ("error out"=w608:errorcluster)  [unwired: 8 in, 1 out]
        n226 = disable-structure shown="Désactivé" {
          disable-tunnel: w608 -> [w631 _]
          disable-tunnel: [w630 _] -> w607
          frame Disabled {
            n227 = Select ("Sélectionner")(t="1", s=FALSE ("sélecteur"), f="0" ("cas faux")) -> (s? t:f=w626:string)
            n228 = local read "BDD"() -> (w629:T2)
            n229 = Bundle By Name(cluster=w629, "Résultat final"=w626) -> (w625:T2)
            n230 = call "BDD_2.vi"("errin"=w631, "Cluster"=w625) -> ("error out"=w630:errorcluster)  [unwired: 8 in, 1 out]
          }
          frame Enabled {
          }
        }
        n231 = flat-sequence {
          tunnel: [TRUE] -> w617
          tunnel: w607 -> [_]
          frame #0 {
          }
        }
      }
      frame "Next" {
        w666 = OP300ZP_state."Null"  # Énum
        w667 = OP300ZP_state."Scan"  # Énum
        # "\\\\forseepower.com\\fr\\040 Production\\FR7 - Poitiers\\06 Production\\05. Electronique\\Documents Control lib\\Archives\\ZEN PLUS"
        n232 = Close File(refnum=w669, error in=w668) -> (path=w650:path, error out=w665:errorcluster)
        n233 = call <userlib>:"waitXms.vi"("attente (ms)"=u32 300, "errin"=w665) -> ("errout"=w660:errorcluster)  [unwired: 13 in]
        n234 = local read "BDD"() -> (w654:T2)
        n235 = Read from Text File(file (use dialog)=w650, error in=w660) -> (text=w659:string, error out=w658:errorcluster)  [unwired: 2 in, 2 out]
        n236 = call "OP300ZP_SN_Reader.vi"("Fichier txt"=w659) -> ("SN"=w638:string)  [unwired: 10 in]
        n237 = Unbundle By Name(w654) -> ("PN"=w653:string)
        n238 = Concatenate Strings(w653, "-SN" ("chaîne"), w638) -> (w651:string)
        n239 = call "Multi_OUI_NON.vi"("errin"=w649, "errinb"=TRUE, "Tableau"=string[] ["SECU", "Next"]) -> ("errout"=w637:errorcluster, "isok?"=w647:bool)  [unwired: 7 in]
        n240 = local read "BDD"() -> (w644:T2)
        n241 = call "OP300ZP_NouveauDossier.vi"("entrée d'erreur (pas d'erreur)"=w658, "Nom du repertoire (PN SN)"=w651, "Network before adding a new folder"=path "\\\\forseepower.com\\fr/040 Production/FR7 - Poitiers/06 Production/05. Electronique/Documents Control lib/Archives/ZEN PLUS" ("chemin de la cible (utiliser une boîte de dialogue)")) -> ("sortie d'erreur"=w657:errorcluster, "Network after adding a new folder"=w655:path)  [unwired: 7 in]
        n242 = flat-sequence {
          tunnel: [w671] -> w636
          tunnel: w637 -> [w671]
          tunnel: [w670] -> w635
          tunnel: w634 -> [w670]
          frame #0 {
            n243 = local read "BDD"() -> (w674:T2)
            n244 = Bundle By Name(cluster=w674, "Résultat final"="1") -> (w672:T2)
            n245 = local write "BDD"(w672) -> ()
          }
        }
        n246 = Copy ("Copier")(8:w657, 10:w655, 11:w650) -> (0:w634:errorcluster)  [unwired: 2 in, 2 out]
        n247 = local read "BDD"() -> (w633:T2)
        n248 = call "PvgeneratorOP300.vi"("errin"=w635, "BDD"=w633, "network"=w655, "path in"=w650) -> ("sortie d'erreur"=w663:errorcluster, "network out"=w662:path, "tout bon"=w661:bool, "chaîne concaténée"=→"chaîne concaténée":string)  [unwired: 3 in, 1 out]
        n249 = Select ("Sélectionner")(t="1", s=w661, f="0" ("cas faux")) -> (s? t:f=w641:string)
        n250 = Bundle By Name(cluster=w644, "Résultat final"=w641, "SN"=w638) -> (w640:T2)
        n251 = local write "BDD"(w640) -> ()
        n252 = call "POP_GOOGLE.vi"("error in"=w663, "chemin"=w662) -> ("error out"=w639:errorcluster)  [unwired: 8 in, 1 out]
        n253 = Select(t=w667, s=w647, f=w666) -> (s? t:f=w645:T6)
      }
      frame "Hydrau" {
        # "A modifier avec hydrau haut"
        n254 = global write "VG_HYDRAU.vi" "CONTI HYDRAU"(0.0 ("R")) -> ()
        n255 = call <userlib>:"OUINON.vi"("errin"=w702, "image"="CONTI_HYDRAU_HAUT" ("IN")) -> ("error out"=w689:errorcluster, "OUI/NON"=w692:bool)  [unwired: 8 in]
        n256 = global read "VG_BT3562.vi" "BT3562"() -> (w688:string)
        n257 = flat-sequence {
          tunnel: w692 -> [w712]
          tunnel: [w711] -> w700
          tunnel: w689 -> [w710]
          tunnel: w688 -> [w709]
          tunnel: [w708] -> w681
          tunnel: [w756] -> w680
          tunnel: [w755] -> w691
          tunnel: [w754] -> w690
          tunnel: w700 -> [w754]
          tunnel: [w753] -> w679
          tunnel: w681 -> [w753]
          frame #0 {
            n258 = case shown="True" w712 {
              tunnel: [w714 w719] -> w711
              tunnel: w710 -> [w714 w717]
              tunnel: w709 -> [_ w716]
              tunnel: [FALSE ("OK?") w715] -> w708
              frame False {
              }
              frame True {
                n259 = while {
                  tunnel: [w739] -> w718
                  tunnel: w717 -> [w733]
                  tunnel: w716 -> [w721]
                  tunnel: [w728] -> w715
                  i -> [w730]
                  stop <- w722 stop-if-true
                  n260 = global read "CheminDeBase.vi" "chemin de base"() -> (w731:path)
                  n261 = global read "VG_HYDRAU.vi" "CONTI HYDRAU"() -> (w734:dbl)
                  n262 = call <userlib>:"ACIR_DCIR_BT3562.vi"("juste R?"=TRUE, "errin"=w733, "chemin de base"=w731, "VISAin"=w721) -> ("errout"=w735:errorcluster, "OK?"=w728:bool, "R"=w737:dbl)  [unwired: 2 in, 3 out]
                  n263 = Equal?(x=FALSE, y=w728) -> (x = y?=w724:bool)
                  n264 = Greater Or Equal?(x=w730, y=2) -> (x >= y?=w725:bool)
                  n265 = case shown="True" w728 {
                    selector: w728 -> [w742 _]
                    tunnel: w735 -> [w740 w744]
                    tunnel: [w740 w746] -> w739
                    tunnel: [w741 "last?"] -> w736
                    tunnel: w730 -> [_ w749]
                    frame False {
                      n266 = Not(x=w742) -> (.not. x?=w741:bool)
                    }
                    frame True {
                      n267 = Add(x=1, y=w749) -> ()  [unwired: 1 out]
                      n268 = call <userlib>:"FGV_Image.vi"("Énum"=FGV."SET", "IN"="2ndBloc") -> ()  [unwired: 9 in, 1 out]
                      n269 = property on="last?" class="Bool"(error in=w744, "Visible"=TRUE) -> (error out=w746:errorcluster)  [unwired: 1 in, 1 out]
                      n270 = Wait (ms)(milliseconds to wait=u32 4000 ("attente (ms)")) -> ()  [unwired: 1 out]
                    }
                  }
                  n271 = Greater Or Equal?(x=w737, y=w734) -> (x >= y?=w738:bool)
                  n272 = And(x=w725, y=w724) -> (x .and. y?=w723:bool)
                  n273 = case shown="True" w738 {
                    tunnel: w737 -> [_ w752]
                    frame False {
                    }
                    frame True {
                      n274 = global write "VG_HYDRAU.vi" "CONTI HYDRAU"(w752) -> ()
                    }
                  }
                  n275 = And(x=w728, y=w736) -> (x .and. y?=w729:bool)
                  n276 = Compound Arithmetic op=OR(w729, w723) -> (w722:bool)
                }
                n277 = property on="last?" class="Bool"(error in=w718, "Visible"=FALSE) -> (error out=w719:errorcluster)  [unwired: 1 in, 1 out]
              }
            }
          }
          frame #1 {
            n278 = call <vilib>:"Application Directory.vi"() -> ()  [unwired: 1 out]
            n279 = global read "VG_HYDRAU.vi" "CONTI HYDRAU"() -> (w755:dbl)
            n280 = call <userlib>:"Read_Param.vi"("Énum"=enum16{"STR", "DBL", "U32"}."DBL", "section"="Conti", "key"="Rmax") -> ("dbl"=w758:dbl)  [unwired: 4 in, 4 out]
            n281 = In Range and Coerce(upper limit=w758, x=w755, lower limit=1.0 ("limite inférieure")) -> (In Range?=w756:bool)  [unwired: 1 out]
          }
        }
        n282 = local write "TOP"("Continuité Blocs hydrauliques haut" ("TOP")) -> ()
        n283 = Number To Decimal String(number=w691) -> (decimal integer string=w696:string)  [unwired: 1 in]
        n284 = Concatenate Strings("Hydrau;" ("chaîne"), w696) -> (w676:string)
        n285 = call "Log_basic.vi"("errin"=w707, "date?"=TRUE, "chaîne"=w676, "in"=w706) -> ("sortie d'erreur"=w703:errorcluster, "refnum en sortie"=w685:refnum<file>)  [unwired: 6 in]
        n286 = And(x=w679, y=w680) -> (x .and. y?=w678:bool)
        n287 = Refnum to Path(1:w685) -> (0:w686:path)
        n288 = local read "BDD"() -> (w698:T2)
        n289 = call "ZenPlusOP300_refaire.vi"("refaire"=w683, "Pédale"=FALSE, "casOK"=OP300ZP_state."Next" ("Cas OK"), "errin"=w690, "test ok ?"=w678) -> ("errout"=w705:errorcluster, "Next"=w701:T6)  [unwired: 5 in]
        n290 = call <userlib>:"TEMPS_TEST.vi"("errin"=w703, "pathin"=w686) -> ("error out"=w687:errorcluster, "Delay calculé"=w684:string)  [unwired: 8 in]
        n291 = Bundle By Name(cluster=w698, "ContiHydrau"=w696, "TempsTest"=w684) -> (w697:T2)
        n292 = local write "BDD"(w697) -> ()
      }
      frame "Sealing" {
        n293 = disable-structure shown="Enabled" {
          disable-tunnel: w770 -> [w785 _]
          disable-tunnel: w769 -> [w780 _]
          disable-tunnel: [w779 _] -> w768
          disable-tunnel: w767 -> [w778 _]
          disable-tunnel: [w777 _] -> w766
          disable-tunnel: w764 -> [w775 _]
          disable-tunnel: [w774 _] -> w763
          disable-tunnel: [w773 _] -> w762
          frame Disabled {
            n294 = call "OP300ZP_SEALING.vi"("ERRIN"=w785) -> ("ERROUT"=w771:errorcluster, "SEALING_VALUE"=w781:dbl, "IsOK?"=w772:bool)  [unwired: 8 in]
            n295 = call "ZenPlusOP300_refaire.vi"("refaire"=w775, "casOK"=OP300ZP_state."Next" ("Cas OK"), "errin"=w771, "test ok ?"=w772) -> ("errout"=w773:errorcluster, "Next"=w774:T6)  [unwired: 6 in]
            n296 = case shown="True" w772 {
              tunnel: w780 -> [w786 w794]
              tunnel: w778 -> [w788 w793]
              tunnel: [w788 w792] -> w777
              tunnel: ["0" w791] -> w782
              tunnel: [w786 w790] -> w779
              tunnel: w781 -> [_ w789]
              frame False {
              }
              frame True {
                n297 = Number To Decimal String(number=w789) -> (decimal integer string=w791:string)  [unwired: 1 in]
                n298 = Concatenate Strings("Sealing;" ("chaîne"), w791) -> (w796:string)
                n299 = call "Log_basic.vi"("errin"=w794, "date?"=TRUE, "chaîne"=w796, "in"=w793) -> ("sortie d'erreur"=w790:errorcluster, "refnum en sortie"=w792:refnum<file>)  [unwired: 6 in]
              }
            }
            n300 = local read "BDD"() -> (w784:T2)
            n301 = Bundle By Name(cluster=w784, "Sealing"=w782) -> (w783:T2)
            n302 = local write "BDD"(w783) -> ()
          }
          frame Enabled {
          }
        }
      }
      frame "Comext" {
        n303 = call <userlib>:"OUINON.vi"("errin"=w803, "image"="Comext" ("IN")) -> ("error out"=w802:errorcluster, "OUI/NON"=w799:bool)  [unwired: 8 in]
        n304 = case shown="True" w799 {
          tunnel: w811 -> [w816 w827]
          tunnel: w810 -> [w815 w826]
          tunnel: [w815 w825] -> w809
          tunnel: [w816 w824] -> w808
          tunnel: [OP300ZP_state."Crash" ("OUT") w823] -> w798
          tunnel: w807 -> [_ w822]
          tunnel: [w813 w821] -> w806
          tunnel: w805 -> [_ _]
          tunnel: w802 -> [w813 w820]
          tunnel: [w814 w819] -> w801
          tunnel: w800 -> [w814 w819]
          frame False {
          }
          frame True {
            w840 = OP300ZP_state."Demontage"  # Énum
            n305 = local read "PN"() -> (w838:string)
            n306 = call <userlib>:"Read_Param.vi"("Énum"=enum16{"STR", "DBL", "U32"}."U32", "errin"=w820, "section"="DataDyn", "key"=w838) -> ("error out"=w833:errorcluster, "U32"=w836:u32)  [unwired: 3 in, 3 out]
            n307 = property on="progression" class="Slide (strict)"(error in=w833, "Visible"=TRUE, "Value"=u8 0 ("progression")) -> (error out=w832:errorcluster)  [unwired: 1 in, 1 out]
            n308 = call <userlib>:"FGV_Image.vi"("Énum"=FGV."SET", "IN"="DataDyn") -> ()  [unwired: 9 in, 1 out]
            n309 = call <userlib>:"SCAN CMU.vi"("errin"=w832, "Nb modules"=w836) -> ("errout"=w849:errorcluster, "# température + #tension OK?"=w844:bool, "Vmin"=w848:dbl, "Vmax"=w847:dbl, "Tmin"=w845:dbl, "Tmax"=w846:dbl)  [unwired: 4 out]
            n310 = call "OP300ZP_Test_DataDyn.vi"("Vcell Max (V)"=w847, "MCU"=w844, "Vcell Min (V)"=w848, "errin"=w849, "Température usine (°C)"=21.0, "Tcell Max (°C)"=w846, "Tcell Min (°C)"=w845) -> ("errout"=w843:errorcluster, "datalog"=w851:string, "pass"=w842:bool)  [unwired: 1 in, 1 out]
            n311 = call "Log_basic.vi"("errin"=w827, "date?"=TRUE, "chaîne"=w851, "in"=w826) -> ("sortie d'erreur"=w824:errorcluster, "refnum en sortie"=w825:refnum<file>)  [unwired: 6 in]
            n312 = call "ZenPlusOP300_refaire.vi"("refaire"=w822, "Pédale"=FALSE, "casOK"=w840, "errin"=w843, "test ok ?"=w842) -> ("errout"=w828:errorcluster, "Next"=w823:T6)  [unwired: 5 in]
            n313 = property on="progression" class="Slide (strict)"(error in=w828, "Visible"=FALSE, "Value"=u8 0 ("progression")) -> (error out=w821:errorcluster)  [unwired: 1 in, 1 out]
          }
        }
      }
      frame "OCV" {
        w883 = OP300ZP_state."Iso" ("Cas OK")
        w875 = enum16{"STR", "DBL", "U32"}."DBL" ("Énum")
        n314 = global read "VG_MX5060.vi" "MX5060"() -> (w852:string)
        n315 = call <userlib>:"FGV_Image.vi"("Énum"=FGV."SET", "IN"="OCV") -> ()  [unwired: 9 in, 1 out]
        n316 = call "OP300ZP_Vout.vi"("errin"=w855, "VISA"=w852) -> ("errout"=w854:errorcluster, "Vout lissée"=w853:dbl)  [unwired: 8 in]
        n317 = global read "IS30%.vi" "VG IS30% ?"() -> (w857:bool)
        n318 = local write "TOP"("Meusure de la tension à vide" ("TOP")) -> ()
        n319 = Select ("Sélectionner")(t="OCV30" ("section"), s=w857, f="OCV70" ("cas faux")) -> (s? t:f=w858:string)
        n320 = call <userlib>:"Read_Param.vi"("Énum"=w875, "errin"=w854, "section"=w858, "key"="OCVmax") -> ("error out"=w877:errorcluster, "dbl"=w874:dbl)  [unwired: 3 in, 3 out]
        n321 = call <userlib>:"Read_Param.vi"("Énum"=w875, "errin"=w877, "section"=w858, "key"="OCVmin") -> ("error out"=w876:errorcluster, "dbl"=w873:dbl)  [unwired: 3 in, 3 out]
        n322 = In Range and Coerce(upper limit=w874, x=w853, lower limit=w873) -> (In Range?=w866:bool)  [unwired: 1 out]
        n323 = local read "BDD"() -> (w864:T2)
        n324 = call "ZenPlusOP300_refaire.vi"("refaire"=w861, "casOK"=w883, "errin"=w876, "test ok ?"=w866) -> ("errout"=w867:errorcluster, "Next"=w856:T6)  [unwired: 6 in]
        n325 = Equal?(x=w856, y=w883) -> (x = y?=w882:bool)
        n326 = case shown="True" w882 {
          tunnel: w870 -> [w886 w892]
          tunnel: [w886 w891] -> w869
          tunnel: w872 -> [w885 w890]
          tunnel: [w885 w889] -> w868
          tunnel: w853 -> [_ w888]
          tunnel: ["0" w887] -> w862
          frame False {
          }
          frame True {
            n327 = Number To Decimal String(number=w888) -> (decimal integer string=w887:string)  [unwired: 1 in]
            n328 = Concatenate Strings("OCV;" ("chaîne"), w887) -> (w894:string)
            n329 = call "Log_basic.vi"("errin"=w892, "date?"=TRUE, "chaîne"=w894, "in"=w890) -> ("sortie d'erreur"=w891:errorcluster, "refnum en sortie"=w889:refnum<file>)  [unwired: 6 in]
          }
        }
        n330 = Bundle By Name(cluster=w864, "OCV"=w862) -> (w863:T2)
        n331 = local write "BDD"(w863) -> ()
      }
    }
    n332 = Wait (ms)(milliseconds to wait=u32 200 ("attente (ms)")) -> ()  [unwired: 1 out]
    n333 = case shown="False" w27 {
      selector: w27 -> [_ w896]
      frame False {
      }
      frame True {
        n334 = local write "STOP"(w896) -> ()
      }
    }
  }
  n335 = while {
    shift-right: [w905] -> _
    shift-left: errorcluster {"status"=FALSE, "code"=0, "source"=""} ("error out") -> [w902]
    stop <- w903 stop-if-true
    # "ici tu met l'image à jour si besoin"
    n336 = Wait (ms)(milliseconds to wait=u32 10 ("attente (ms)")) -> ()  [unwired: 1 out]
    n337 = call <userlib>:"FGV_Image.vi"("Énum"=FGV."GET") -> ("OUT"=w898:string)  [unwired: 10 in]
    n338 = Not Equal?(x=w898, y="") -> (x != y?=w899:bool)
    n339 = case shown="False" w899 {
      tunnel: [w907 w912] -> w905
      tunnel: w902 -> [w907 w911]
      tunnel: w898 -> [_ w910]
      frame False {
      }
      frame True {
        n340 = call <vilib>:"Application Directory.vi"() -> ("Application Directory"=w915:path)
        n341 = Path To String(path=w915) -> (string=w916:string)
        n342 = Concatenate Strings(w916, "\\Image\\" ("chaîne"), w910, ".jpg" ("chaîne")) -> (w914:string)
        n343 = call <userlib>:"FGV_Image.vi"("Énum"=FGV."RAZ") -> ()  [unwired: 10 in, 1 out]
        n344 = String To Path(string=w914) -> (path=w913:path)
        n345 = call <vilib>:"Read JPEG File.vi"("error in (no error)"=w911, "path to JPEG file"=w913) -> ("error out"=w912:errorcluster, "image data"=w919:T10)  [unwired: 7 in, 1 out]
        n346 = call <vilib>:"Draw Flattened Pixmap.vi"("image data"=w919) -> ("new picture"=w908:picture)  [unwired: 8 in]
        n347 = local write "DRAW"(w908) -> ()
      }
    }
    n348 = global read "VG_progressBar.vi" "progression"() -> (→"progression":dbl)
    n349 = local read "STOP"() -> (w904:bool)
    n350 = Or(x=w905, y=w904) -> (x .or. y?=w903:bool)
  }
  n351 = while {
    tunnel: [w921] -> w3
    shift-right: [w920] -> _
    shift-left: errorcluster {"status"=FALSE, "code"=0, "source"=""} ("error out") -> [w920]
    stop <- w921 stop-if-true
    n352 = call "ARRET.vi"("arrêt"="arrêt") -> ("T button?"=w921:bool)  [unwired: 10 in]
  }
  n353 = Stop(stop? (T)=w3) -> ()
  n354 = Merge Errors(w19, w18) -> (→"errout":errorcluster)
  n355 = disable-structure shown="Activé" {
    disable-tunnel: [w923 _] -> _
    frame Disabled {
      n356 = call "Data Dynamiques"() -> ("CMU OK"=w923:bool)  [unwired: 12 in, 7 out]
    }
    frame Enabled {
    }
  }
  "STOP" <- w16
